vi "UI.vi"(0 "reference in":refnum<class "GUI Test Channels.lvclass">, 5 "error in (no error)":errorcluster) -> (14 "reference out":refnum<class "GUI Test Channels.lvclass">, 19 "error out":errorcluster)   [LabVIEW 2019, in "GUI Test Channels.lvclass"]
uses:
  GUI Test Channels.lvclass
  C:/Users/ANENKOV_V1/Desktop/src/GUI_class/GUI.lvclass
  FPGA/TypeDef/valveState.ctl
  GUI_class/GUI.lvclass/GUI.ctl
  TypeDef/AI_Data_Array.ctl
  TypeDef/AI_Data.ctl
  TypeDef/AI Statistics Data.ctl
  TypeDef/CalibrationData.ctl
  TypeDef/GUI Setting Channel.ctl
  TypeDef/GUI AI Ranges.ctl
  TypeDef/Scale Data.ctl
  SV_Wrap/SharedVariableWrapper.lvclass/SharedVariableWrapper.ctl
  GUI_class/WindowsState.ctl
  Modbus_class/CMD REG.ctl
  MessageAMC_class/MessageAMC.lvclass
  C:/Users/ANENKOV_V1/Desktop/src/MessageInterface_class/MessageInterface.lvclass
  147e0478-b1e0-44e5-9d90-55d61f62186e.vi
  3e1616dc-8ade-4f65-a997-ed519c35ad68.vi
  1b4fed76-272f-4eb9-b435-1b7916789d73.vi
  d0ca9bf2-7cd9-4c29-a03d-de1c10393a74.vi
  00986001-a254-421c-85fc-d87d850abbb1.vi
  b472a263-1974-420a-8762-279f74d744f3.vi
  7d6317b3-a4cc-487a-a191-d3b197fe0ad7.vi
  7b67f280-2cf4-4c83-93bd-a4bebb40b904.vi
  89ddd393-c331-4ab8-9870-c63a9689f0e3.vi
  816f4990-c02c-40e3-a8e1-ec1953188256.vi
  6ecfee0b-d9cc-4678-92a9-30749ce547e6.vi
  770577dd-3d58-4cb1-b26a-92b56a3dc732.vi
  e7cb1b03-de9d-4d10-b03f-ed147f3d7f4d.vi
  4124e316-6eb4-42ff-9d4a-b566f3345d57.vi
  b80a7f44-ff74-4897-ae94-348c9bf1cb3c.vi
  666d2444-51b8-4c74-bb7d-b80a48b6443e.vi
  GUI_class/Set Win State.vi
  147e0478-b1e0-44e5-9d90-55d61f62186e.vi/52dffe28-1cd0-4ae0-8363-fbbc473a3346.vi
  SV_Wrap/Write Var Info.vi
  SV_Wrap/Read Var Info.vi
  1b4fed76-272f-4eb9-b435-1b7916789d73.vi/5389994d-5541-411f-974c-94a5d08bd79d.vi
  d0ca9bf2-7cd9-4c29-a03d-de1c10393a74.vi/e242b2b1-b066-4fef-9774-8e1a54e29692.vi
  00986001-a254-421c-85fc-d87d850abbb1.vi/269d6d4e-e5f8-46fa-b5a0-5745950f586b.vi
  b472a263-1974-420a-8762-279f74d744f3.vi/f9a62cb2-ec71-4724-a147-a33e2b02a7cc.vi
  7d6317b3-a4cc-487a-a191-d3b197fe0ad7.vi/0852bef6-d0ca-4adc-9038-96861f44a805.vi
  7b67f280-2cf4-4c83-93bd-a4bebb40b904.vi/a928b4cf-f8d6-4ce5-931e-e4c32b09a882.vi
  89ddd393-c331-4ab8-9870-c63a9689f0e3.vi/67eb750a-c2db-4242-8b04-f1964937678c.vi
  e7cb1b03-de9d-4d10-b03f-ed147f3d7f4d.vi/e2f146e0-dd5e-45e4-842e-c2408875ec0c.vi
  SV_Wrap/Read connection str.vi
  <userlib>/_OpenG.lib/time/time.llb/Tick Count (ms)__ogtk.vi
  GUI_class/GUI.lvclass
  MessageInterface_class/MessageInterface.lvclass
  SV_Wrap/SharedVariableWrapper.lvclass
panel:
  out "CHMBR":cluster{"scl mean 1Hz":dbl, "scl mean":dbl}(graph) caption="Давление в камере [МПа]"
  out "DUT":cluster{"scl mean 1Hz":dbl, "scl mean":dbl}(graph) caption="Давление в образце [МПа]"
  out "P_CHMBR_MB":dbl caption="MB" format="%.2f"
  out "P_DUT_MB":dbl caption="MB" format="%.2f"
  in  "=0":bool
  in  "-0,1":bool
  in  "+0,1":bool
  in  "alarm press":bool
  out "data out 2":T1
  out "data out":T1
  out "AI4":dbl(slide) caption="AI 4" scale=0.0..1.0
  out "AI1":dbl(slide) caption="Температура [AI1]" scale=0.0..100.0
  out "AI3":dbl(slide)=57.25190839694657 caption="Температура [AI3]" scale=0.0..100.0
  out "AI_2":dbl(slide)=57.25190839694657 caption="Уровень [AI2]" scale=0.0..100.0
  out "AI_0":dbl(slide)=57.25190839694657 caption="Уровень [AI0]" scale=0.0..100.0
  in  "DO 25":bool caption="Stop SD [37.2]"
  in  "DO 24":bool caption="Stop SD [37.1]"
  out "DI 30":bool caption="44.2 закрыт"
  out "DI 29":bool caption="44.2 открыт"
  out "DI 22":bool caption="44.1 закрыт"
  out "DI 21":bool caption="44.1 открыт"
  in  "DO 23":bool caption="KP24 Y44.2 抢市."
  in  "DO 22":bool caption="KP23 Y44.2 ОТК."
  in  "DO 21":bool caption="KP22 Y44.1 抢市."
  in  "DO 20":bool caption="KP21 Y44.1 ОТК."
  in  "DO 19":bool caption="Драйверы KP20"
  in  "DO 17":bool caption="KP18 Y29.13 33.3"
  in  "DO 18":bool caption="Подача воздук KP19"
  out "DI 11":bool caption="Состояние БП [G2]"
  out "DI 20":bool caption="Фильтр [S4]"
  out "DI 19":bool caption="Фильтр [S3]"
  out "DI 18":bool caption="Фильтр [S2]"
  out "DI 17":bool caption="Фильтр [S1]"
  out "DI 8":bool caption="QF9"
  out "DI 7":bool caption="QF8"
  out "DI 6":bool caption="QF7"
  out "DI 5":bool caption="QF6"
  out "Connect":bool caption="Подключение"
  in  "Reset Alarms":bool
  in  "stop":bool
  out "DI 10":bool caption="Состояние БП [G1]"
  out "DI 9":bool caption="Реле контроля фаз, контактор [KV1]"
  out "DI 4":bool caption="QF5"
  out "DI 3":bool caption="QF4"
  out "DI 2":bool caption="QF3"
  out "DI 1":bool caption="QF2"
  out "DI 0":bool caption="QF1"
  out "DI 26":bool caption="Автомат [QF12]"
  out "DI 25":bool caption="Контактор [MK2]"
  out "DI 28":bool caption="Автомат [QF13]"
  out "DI 27":bool caption="Контактор [MK3]"
  out "DI 24":bool caption="Автомат [QF11]"
  out "DI 23":bool caption="Контактор [MK1]"
  in  "AO 1":dbl(slide) caption="AO 0" scale=0.0..10.0
  in  "AO 0":dbl(slide) min=0.0 max=2.0 step=0.01 scale=0.0..1.0 scale format="%#.2f"
  in  "DO 16":bool caption="KP17 Y29.12  33.4"
  in  "DO 15":bool caption="KP16 Y29.11  33.5"
  in  "DO 14":bool caption="KP15 Y29.10  33.6"
  in  "DO 13":bool caption="KP14 Y29.9 33.10"
  in  "DO 12":bool caption="KP13 Y29.8  33.11"
  in  "DO 11":bool caption="KP12 Y29.7  33.13"
  in  "DO 10":bool caption="KP11 Y29.6 33.2"
  in  "DO 9":bool caption="KP10 Y29.5 33.1"
  in  "DO 8":bool caption="KP9 Y29.4  33.12"
  in  "DO 7":bool caption="KP8 Y29.3 33.9"
  in  "DO 6":bool caption="KP7 Y29.2 33.8"
  in  "DO 5":bool caption="KP6 Y29.1 33.7"
  in  "DO 4":bool caption="Вода Y18.2 [DO4]"
  in  "DO 3":bool caption="Вода Y18.1 [DO3]"
  in  "DO 2":bool caption="Пуск KP3 [DO 2]"
  in  "DO 1":bool caption="Пуск KP2 [DO 1]"
  in  "DO 0":bool caption="Пуск KP1 [DO 0]"
  out "DI 16":bool caption="Переключатель ручное/авто SA1"
  out "DI 15":bool caption="Кнопка аварийной остановки [SB4]"
  out "DI 14":bool caption="Кнопка остановки [SB3]"
  out "DI 13":bool caption="Кнопка запуска [SB2]"
  out "DI 12":bool caption="Кнопка сброса ошибки [SB1]"
  out "AI 10":dbl(knob) caption="Датчик давления в линии \nизмерения утечек  [бар]" scale=0.0..400.0
  out "AI 9":dbl(knob) caption="Давление  в  линии подачи \nвоздуха после БПВ [бар]" scale=0.0..16.0
  out "AI 8":dbl(knob) caption="Давление  в  линии подачи \nвоздуха в БПВ  [бар]" scale=0.0..16.0
  out "AI 7":dbl(knob) caption="Давление в камере [МПа]" scale=0.0..400.0
  out "AI 6":dbl(knob) caption="Давление в образце [МПа]" scale=0.0..400.0
  out "AI 5":dbl(knob) caption="Давление после насоса ВД [МПа]" scale=0.0..400.0
  # "Проверка каналов"
  # "Панель гидравлическая"
  # "Кнопки"
  # "Реле"
  # "Гидростанция очистки и охлаждения [M24]"
  # "Насос перекачки \nв бак подачи [M12]"
  # "Автоматы"
  # "Гидростанция подачи масла [M21]"
  # "Управление  подачей давления в насос ВД"
  # "Регулировка низкого давления в линии подачи масла в насос ВД и напрямую в узел образца"
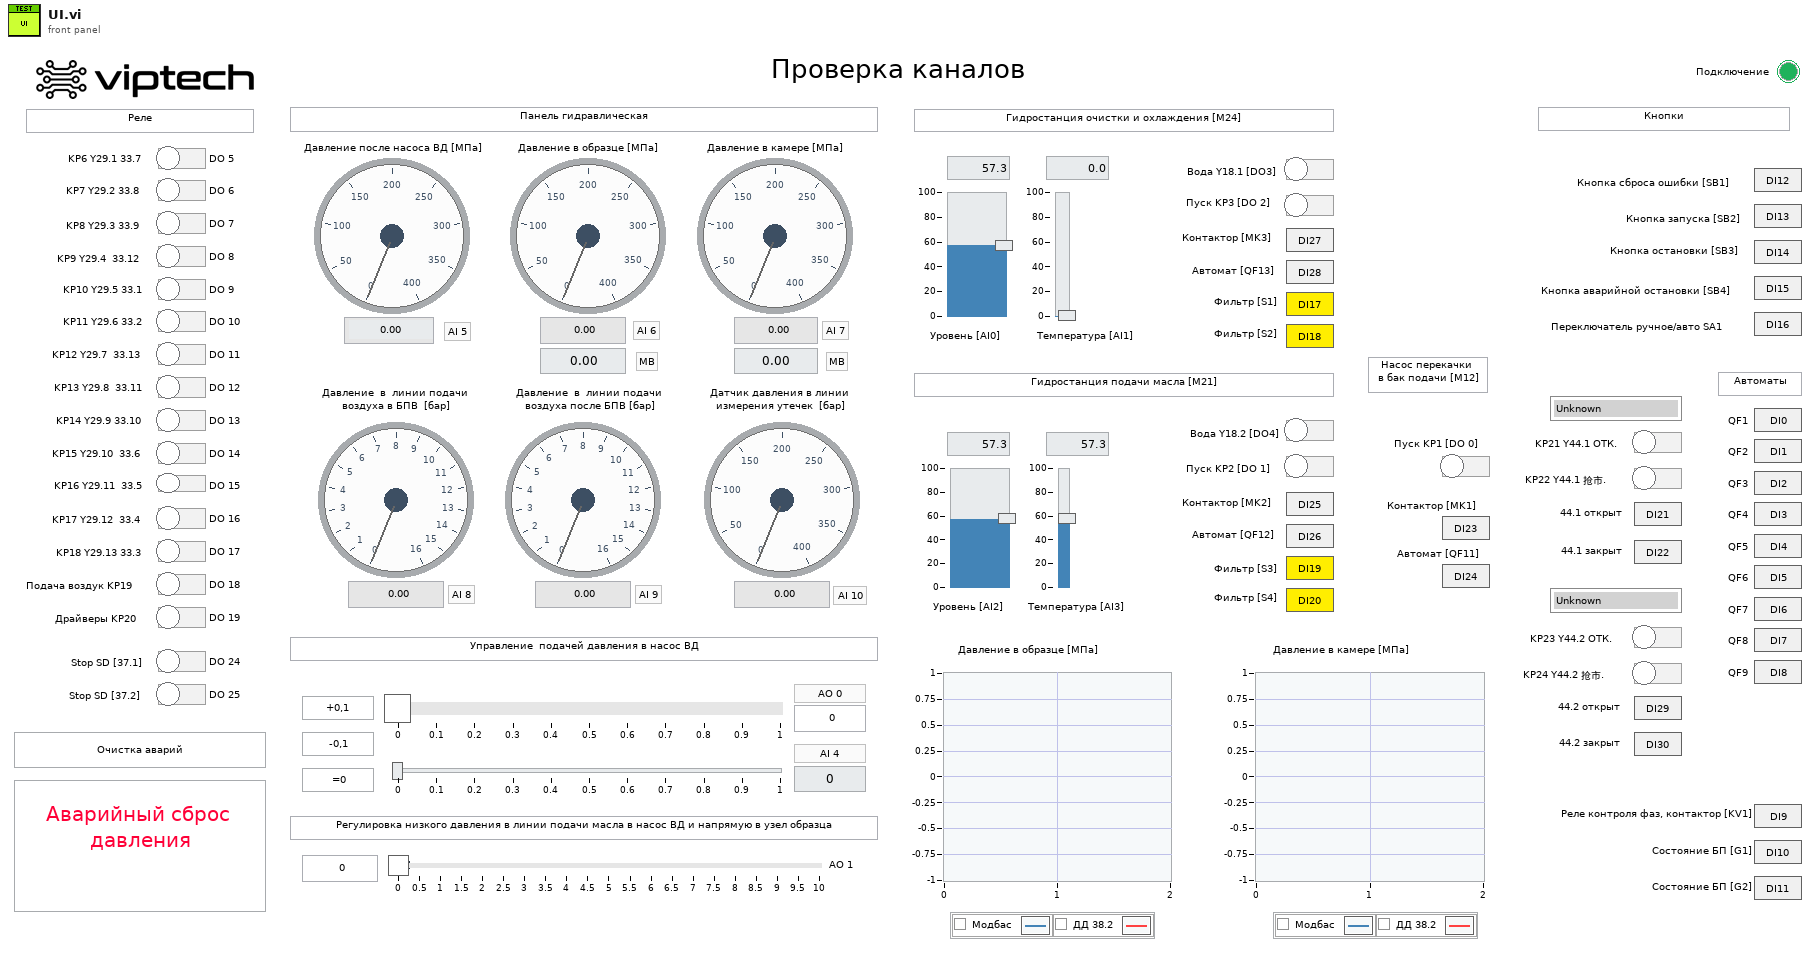
[diagram p1: front panel]
types:
  T1 = typedef "valveState.ctl" = enum16{"Unknown", "Closed", "Opening", "Opened", "Closing"}
  T2 = typedef "CMD REG.ctl" = cluster{"EXECUTE_SP":bool, "ALARM_PRESS_DOWN_DUT":bool, "ALARM_PRESS_DOWN_CHAMBER":bool, "ALARM_PRESS_DOWN_DUT_CHAMBER":bool, "FILING_DUT":bool, "FILING_CHAMBER":bool, "BLOCK":bool, "PUMP_STATION_OFF":bool, "Leak start":bool, "Leak stop":bool, "Drain":bool}
  T3 = enum32{"Invalid", "Standard", "Closed", "Hidden", "Minimized", "Maximized"}
  T4 = enum32{"invalid app kind", "Development System", "Run Time System", "Student Edition", "Embedded LabVIEW", "Evaluation", "Custom"}
  T5 = typedef "SharedVariableWrapper.lvclass/Config.ctl" = cluster{"connection str":string, "timeout":dbl, "ip":string}
  T6 = cluster{"Core":cluster{"Current VI Reference":refnum<vi>, "Close Panel on Exit?":bool}, "amc":refnum<class "MessageAMC.lvclass">}
  T7 = cluster{"Current VI Reference":refnum<vi>, "Close Panel on Exit?":bool}
  T8 = typedef "CalibrationData.ctl" = cluster{"Channels":T9[], "Scales":T11[]}
  T9 = typedef "GUI Setting Channel.ctl" = cluster{"Name":string, "AI Ranges":T10, "ScaleIndex":u32}
  T10 = typedef "GUI AI Ranges.ctl" = cluster{"HI":bool, "HIHI":bool, "LO":bool, "LOLO":bool, "HIHI VAL":dbl, "HI VAL":dbl, "LO VAL":dbl, "LOLO VAL":dbl, "MAX RAW":dbl, "MIN RAW":dbl, "MAX SCALED":dbl, "MIN SCALED":dbl}
  T11 = typedef "Scale Data.ctl" = cluster{"index":i32, "Name":string, "X":dbl[], "Y":dbl[]}
  T12 = typedef "AI_Data_Array.ctl" = T13[]
  T13 = typedef "AI_Data.ctl" = cluster{"Stat Data":T14, "OutOfRangeMax":bool, "OutOfRangeMin":bool, "HIHI":bool, "HI":bool, "LO":bool, "LOLO":bool}
  T14 = typedef "AI Statistics Data.ctl" = cluster{"raw mean":dbl, "scl mean":dbl, "raw mean 1Hz":dbl, "scl mean 1Hz":dbl}
  T15 = typedef "GUI.lvclass/WindowsState.ctl" = enum16{"NotReady", "Ready", "Inserted", "Opened"}
  T16 = typedef "GUI.lvclass/Shered Data.ctl" = cluster{"WindowsState":T15, "UI VI":refnum<vi>, "SubPnl":refnum<vi>}
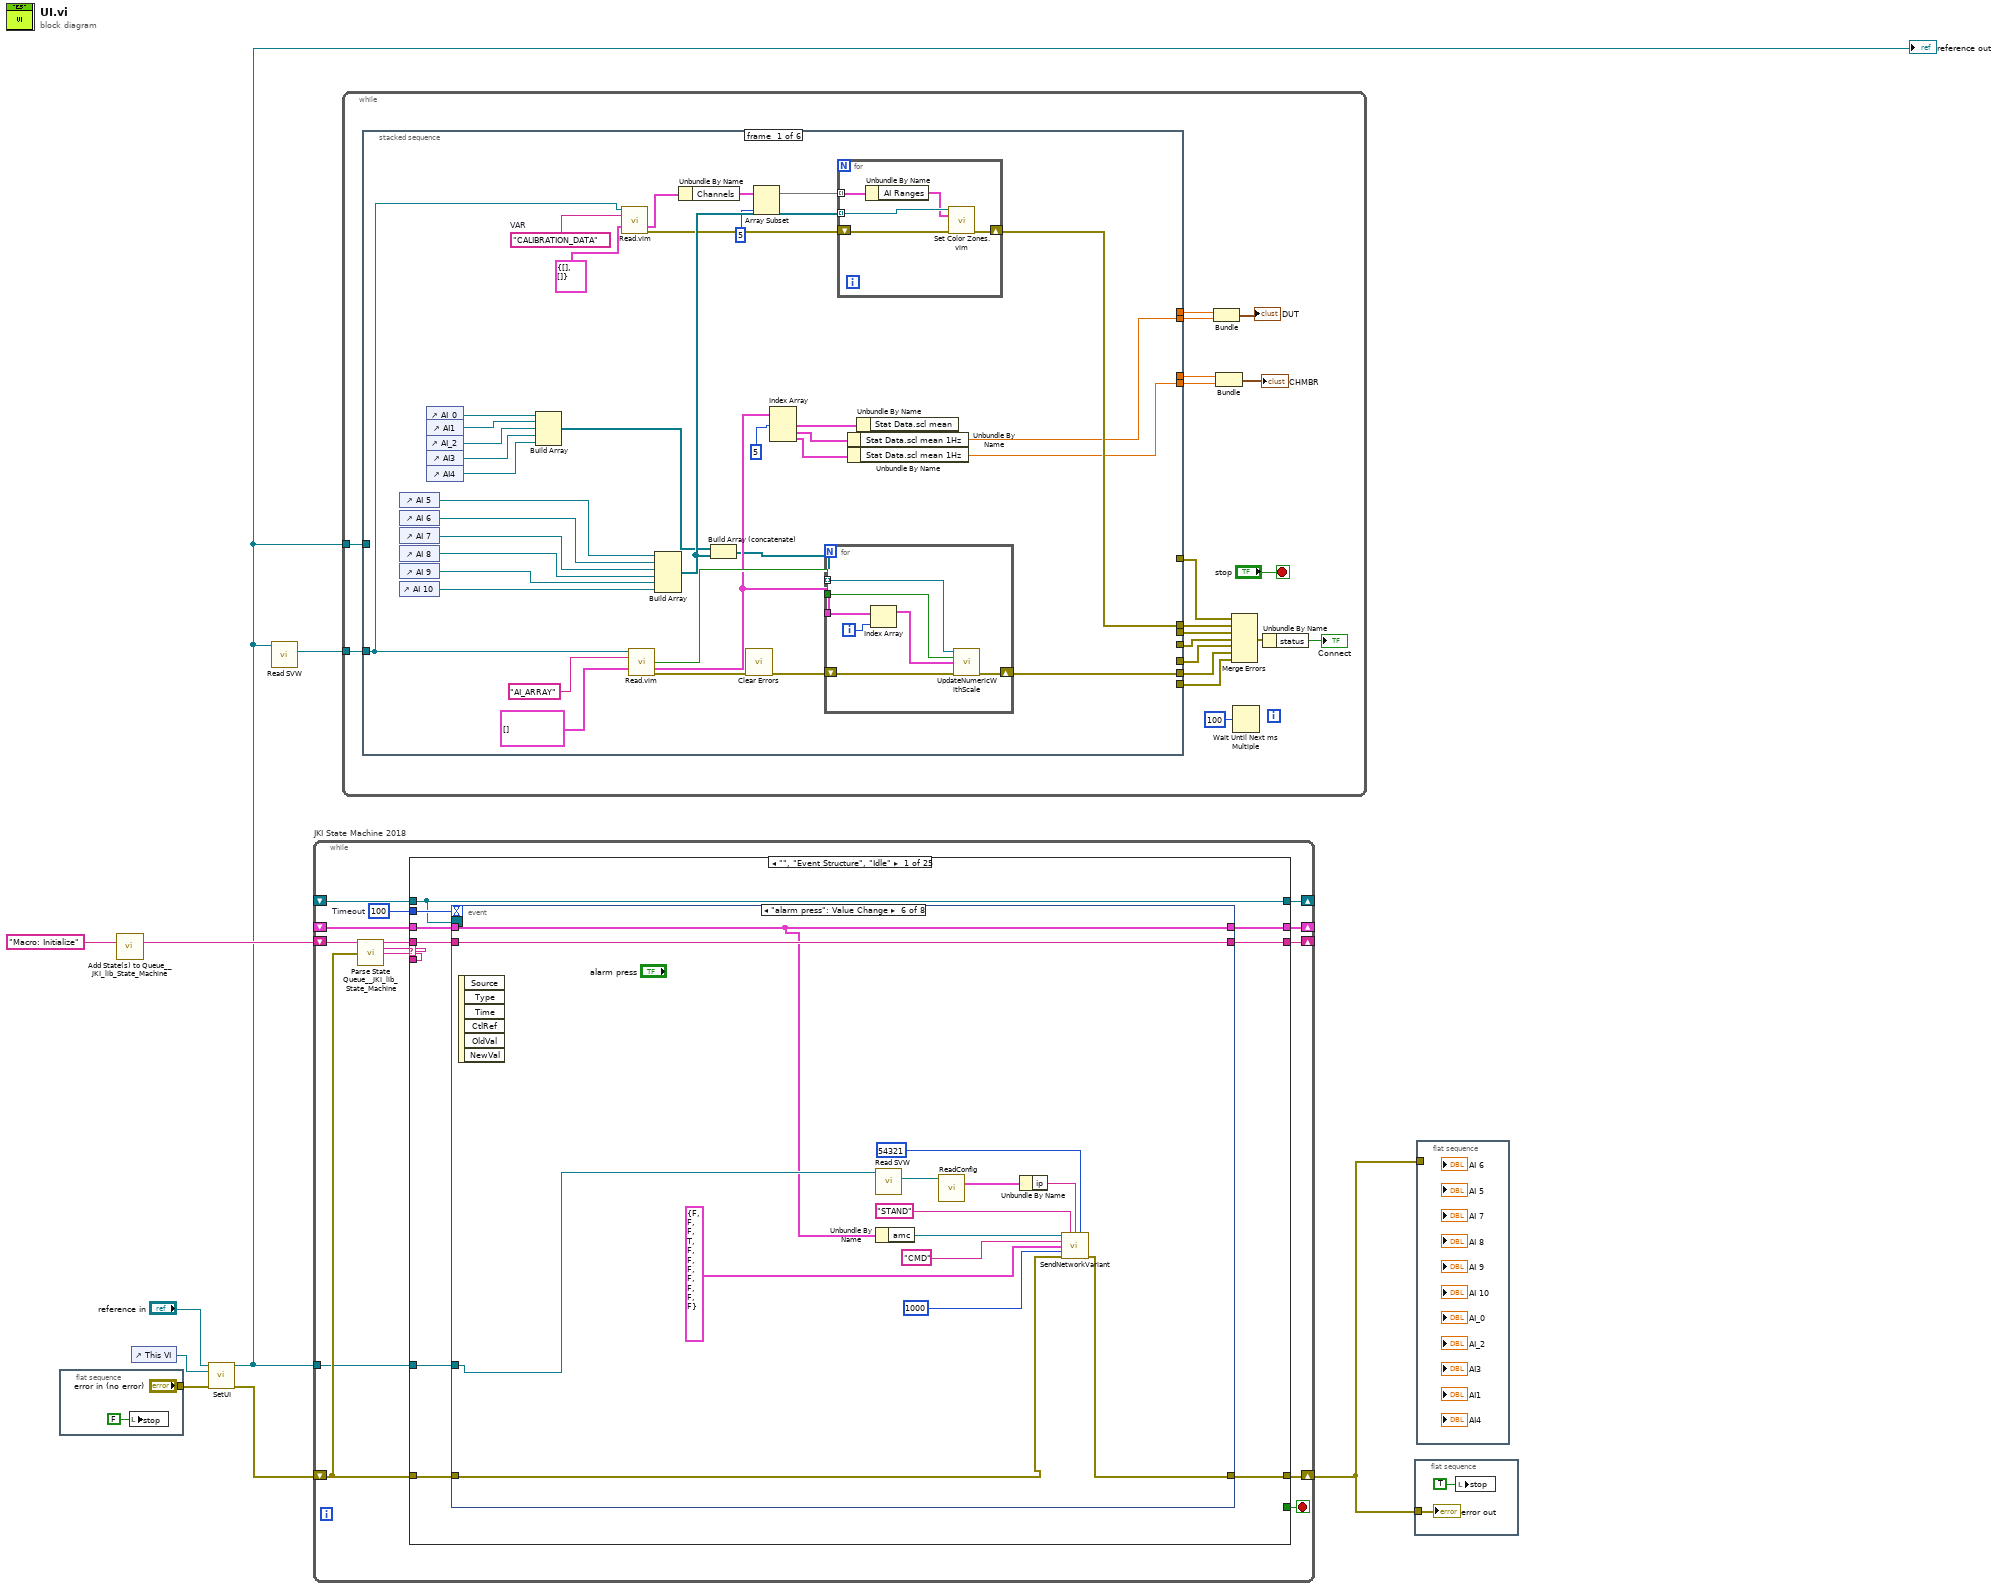
[diagram p0: block diagram]
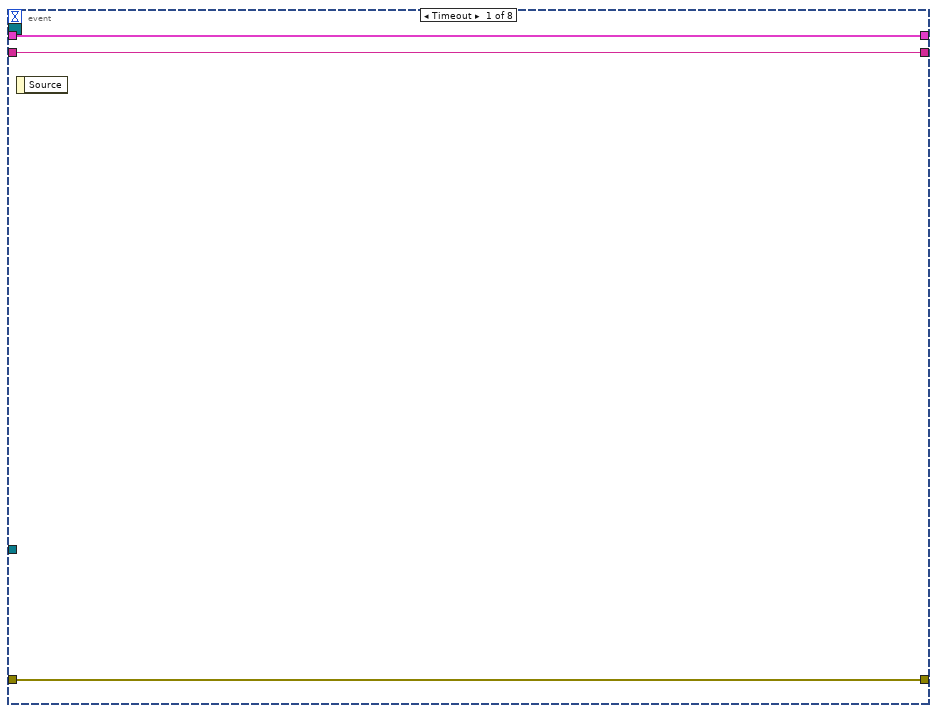
[diagram p2: hidden frame]
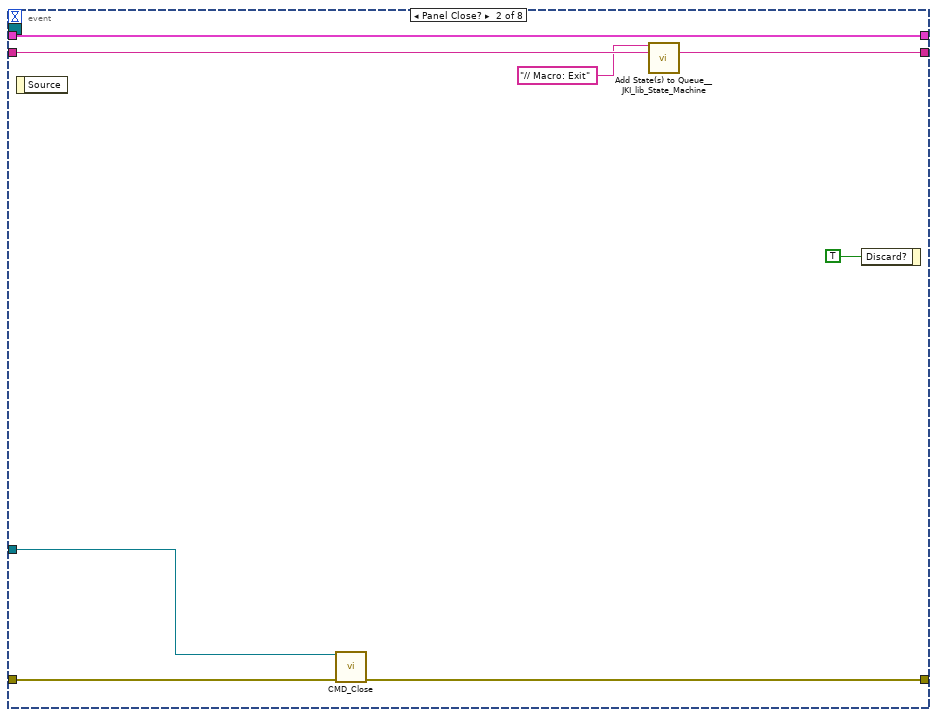
[diagram p3: hidden frame]
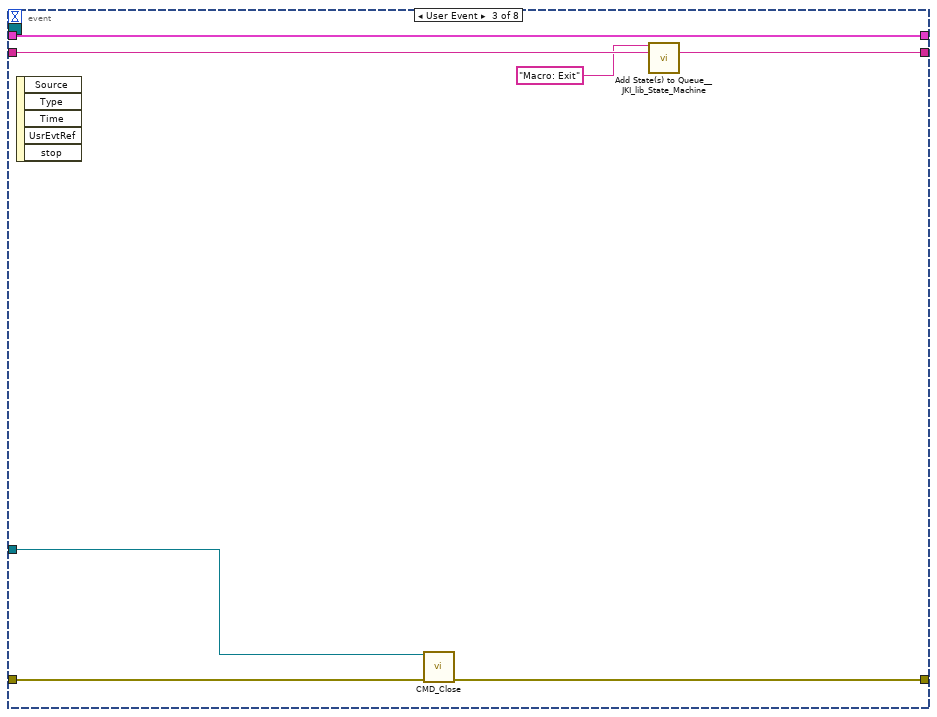
[diagram p4: hidden frame]
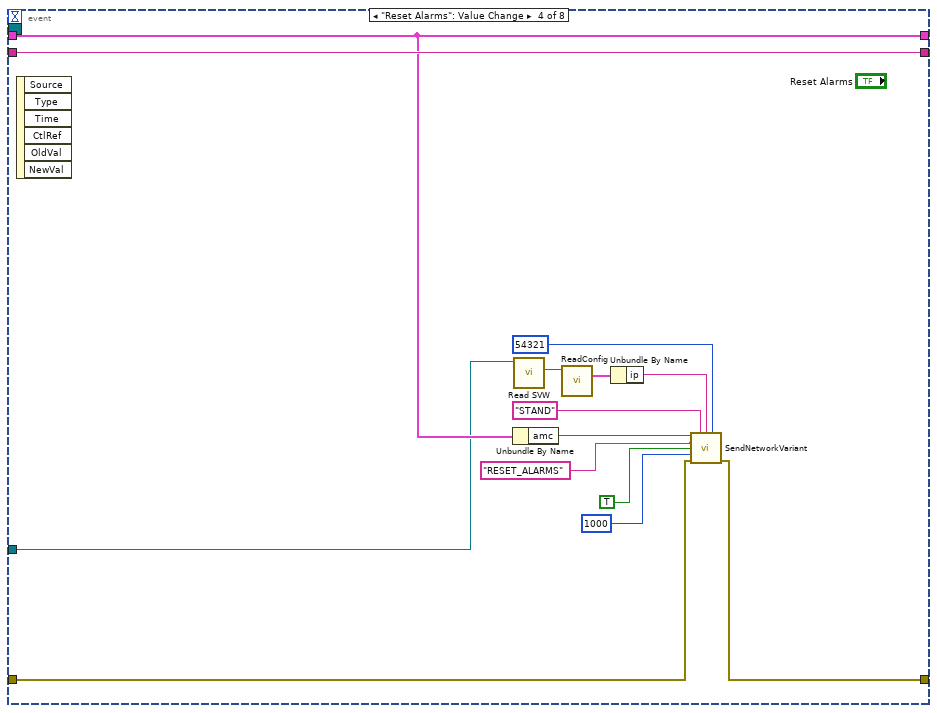
[diagram p5: hidden frame]
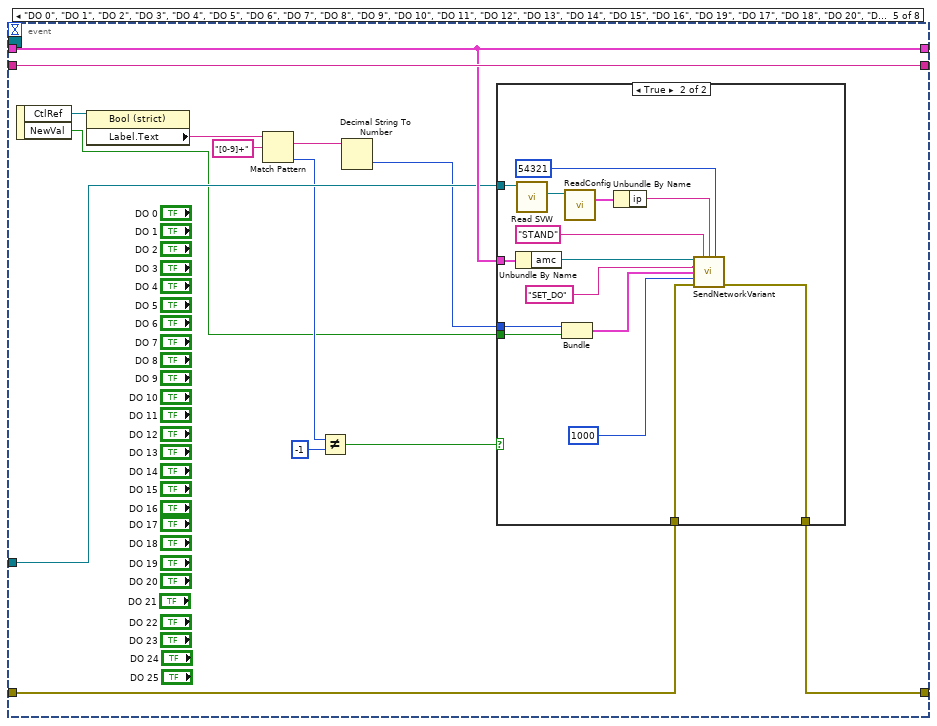
[diagram p6: hidden frame]
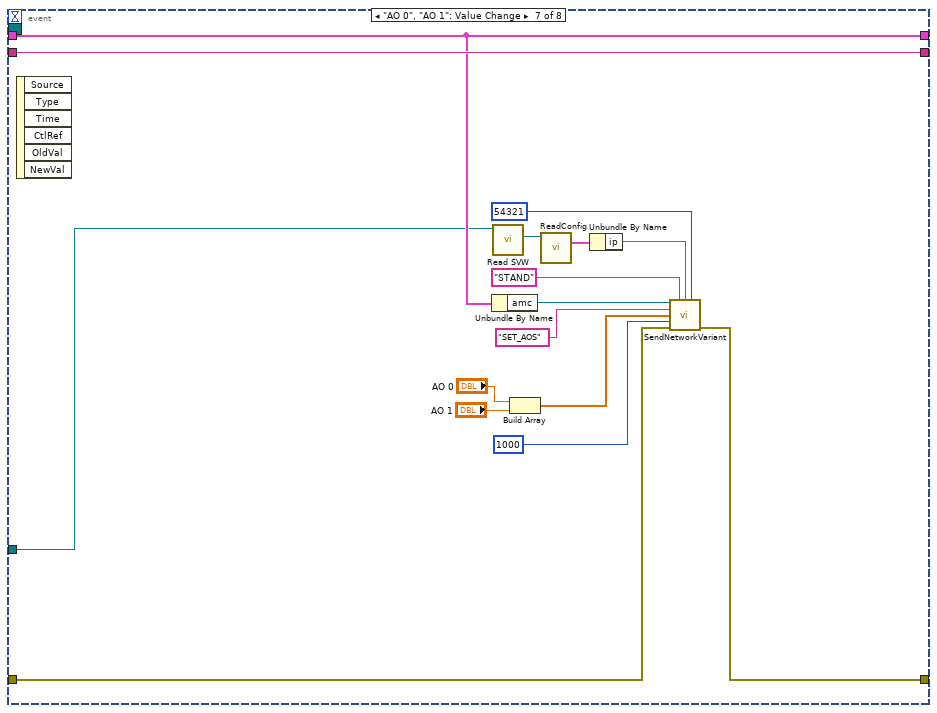
[diagram p8: hidden frame]
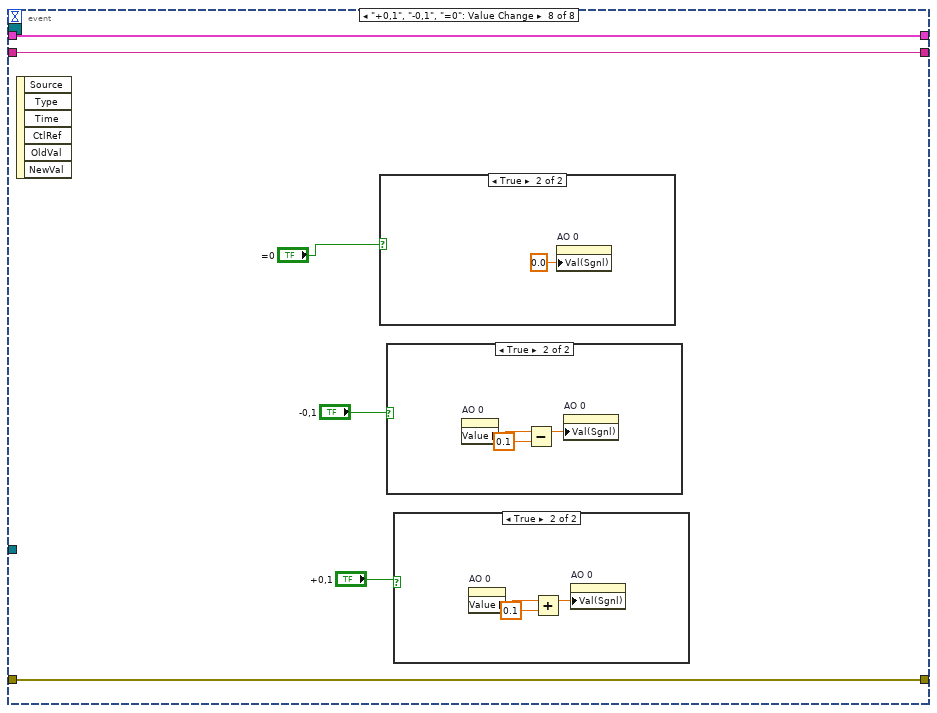
[diagram p9: hidden frame]
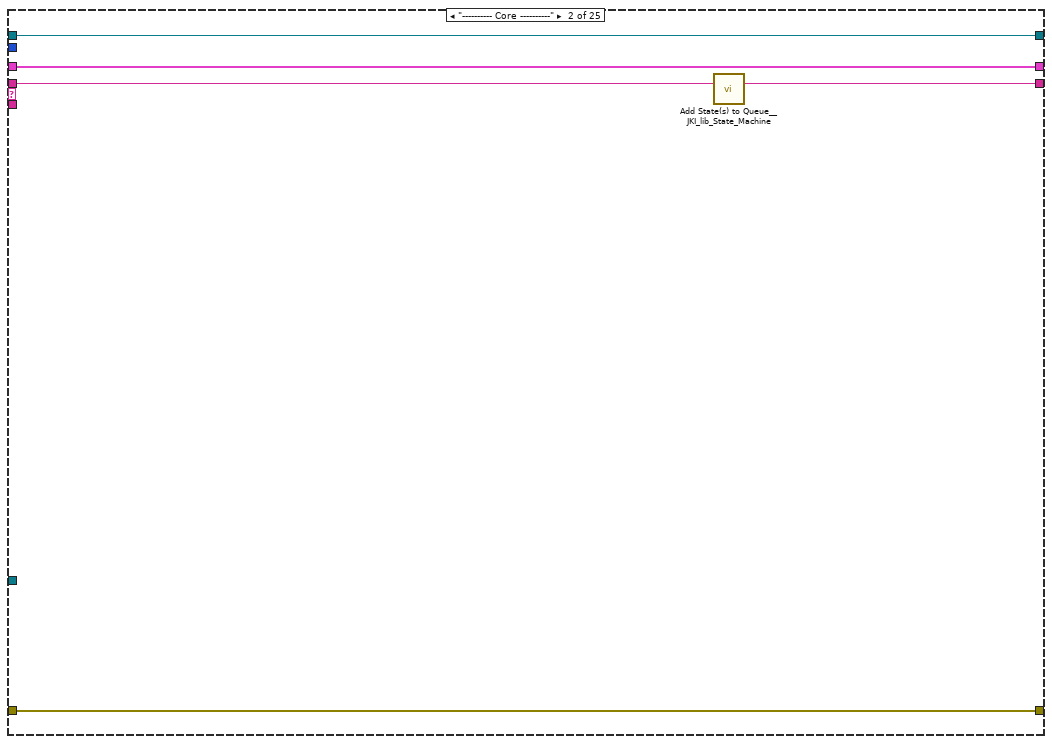
[diagram p13: hidden frame]
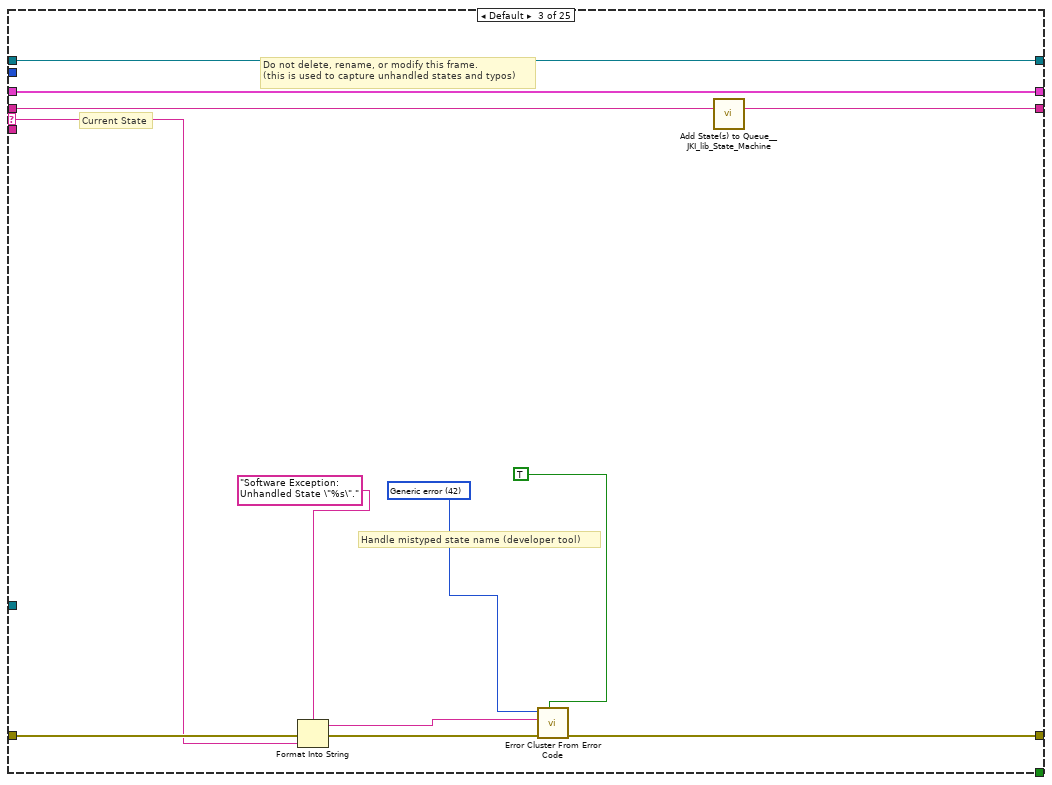
[diagram p14: hidden frame]
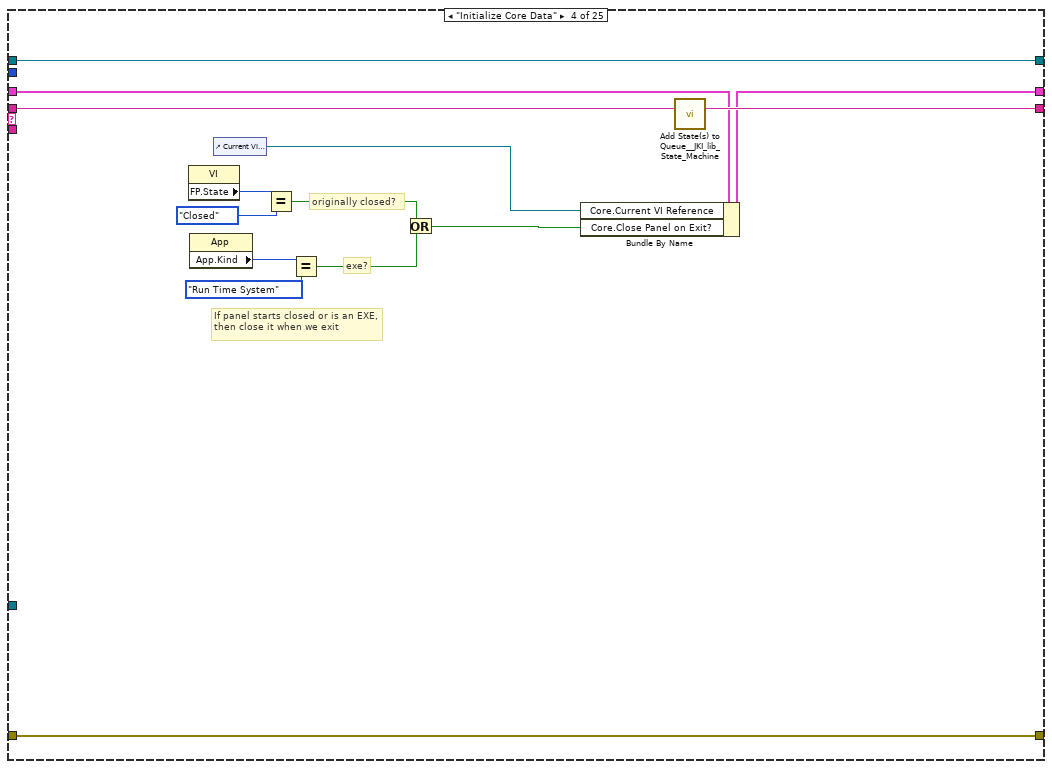
[diagram p15: hidden frame]
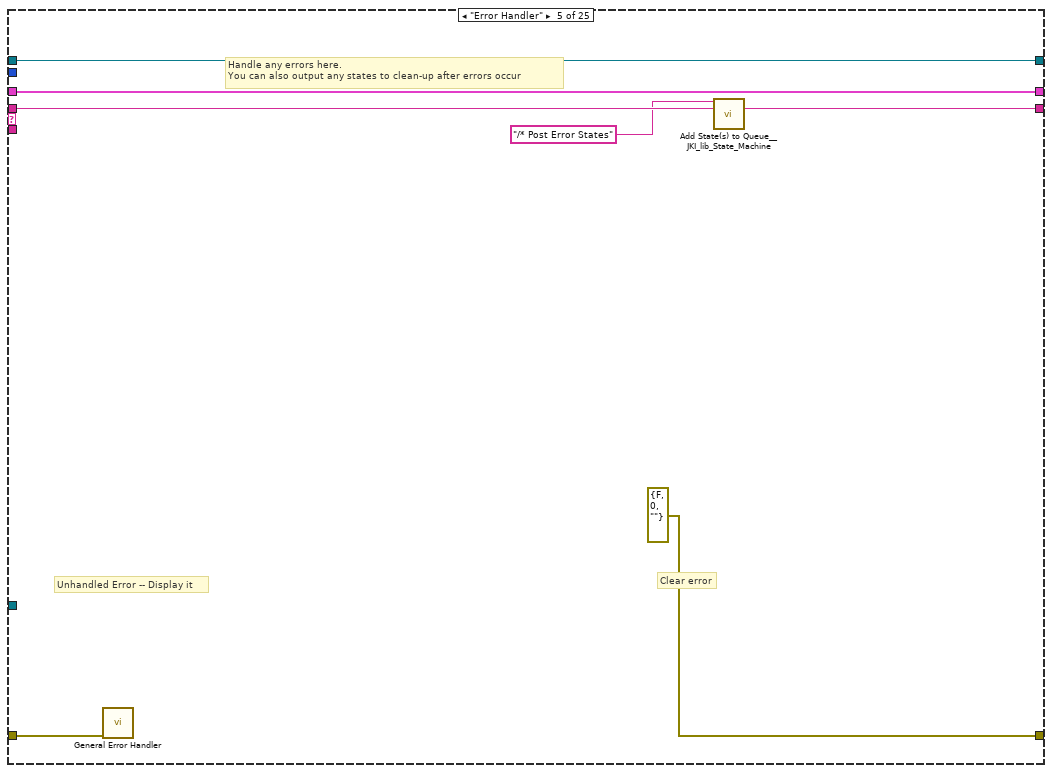
[diagram p16: hidden frame]
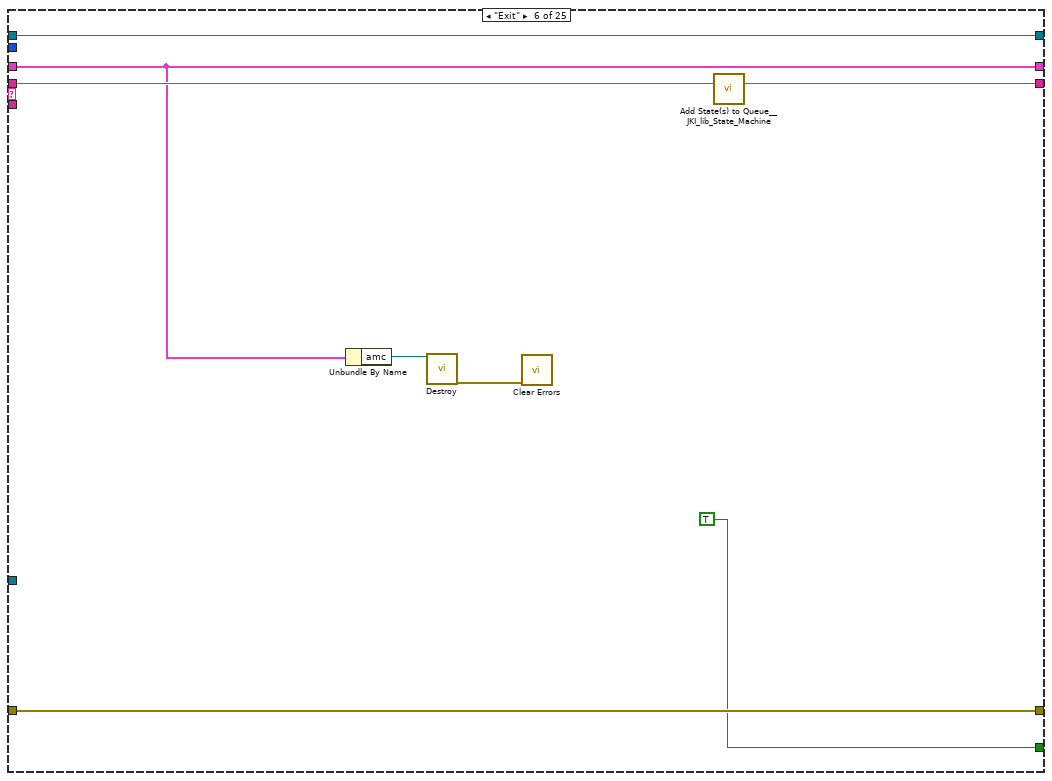
[diagram p17: hidden frame]
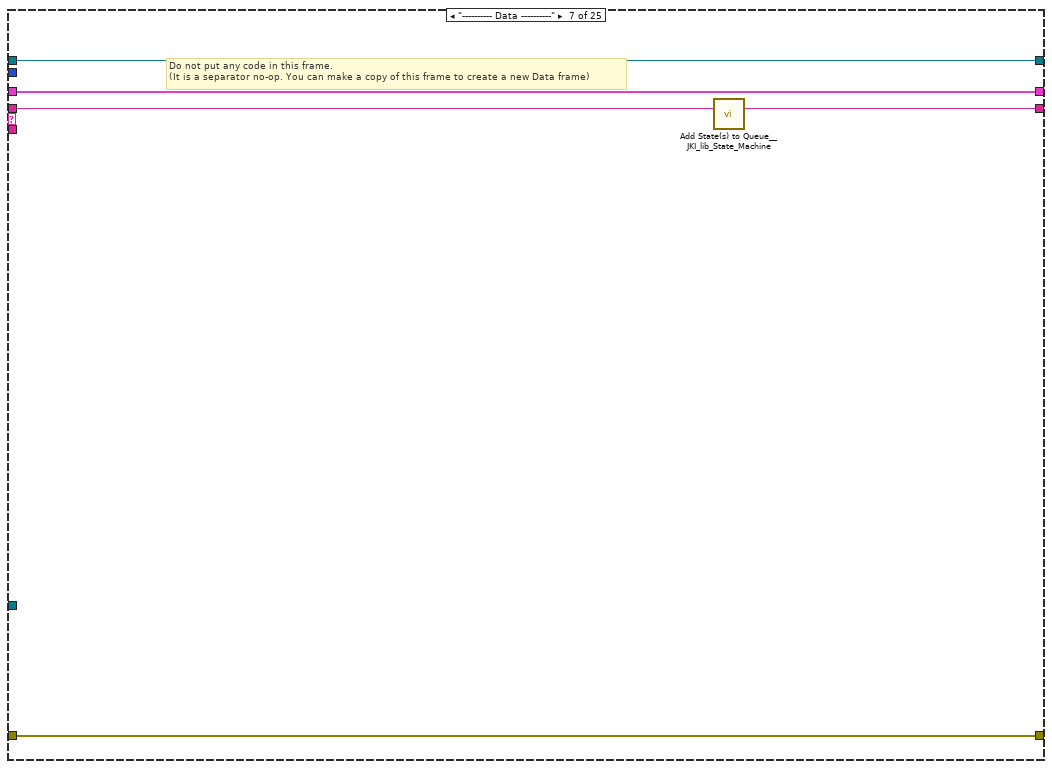
[diagram p18: hidden frame]
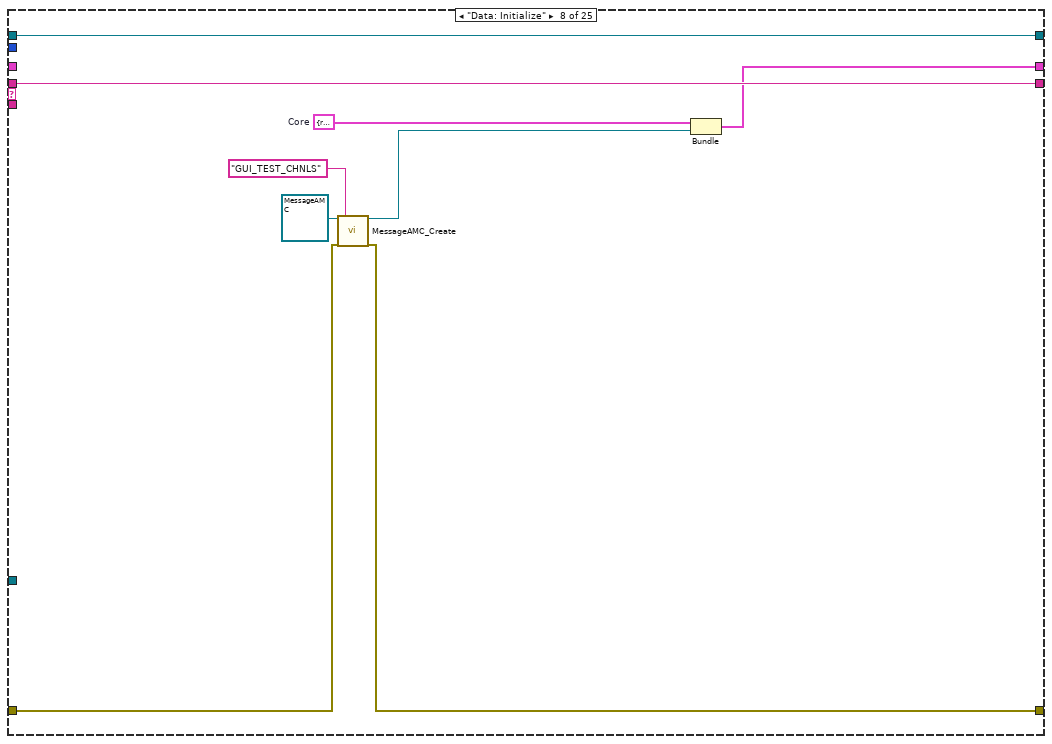
[diagram p19: hidden frame]
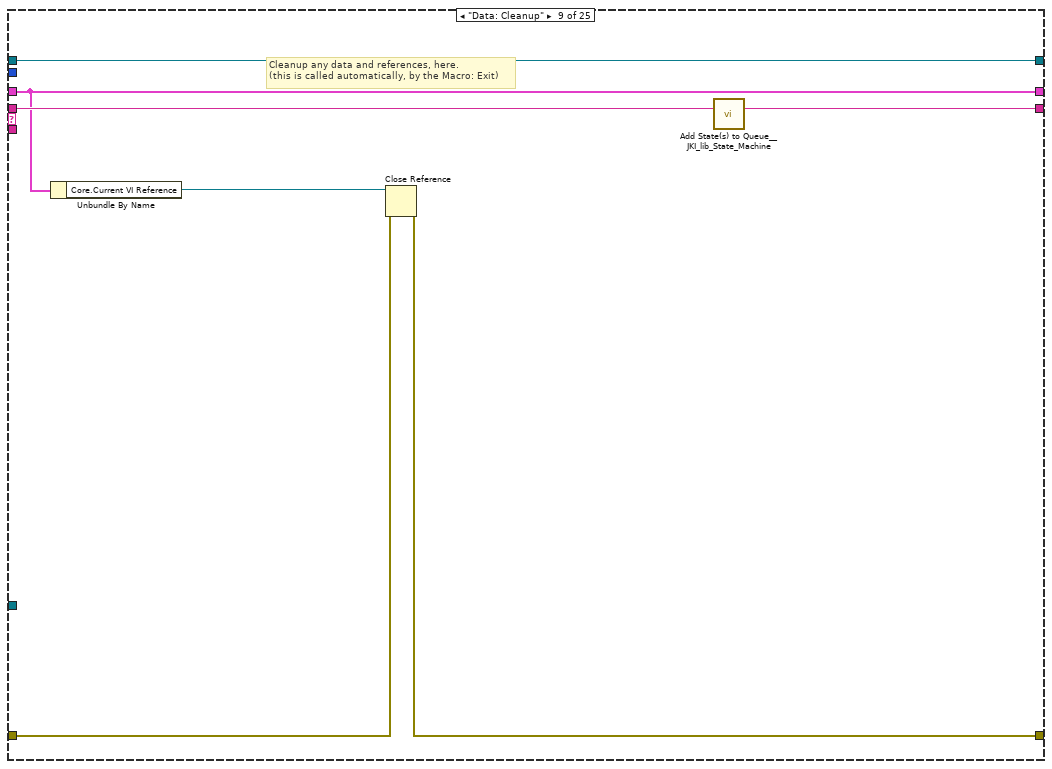
[diagram p20: hidden frame]
diagram:
  n1 = flat-sequence {
    tunnel: ["error in (no error)"] -> w7
    frame #0 {
      n2 = local write "stop"(FALSE ("stop")) -> ()
    }
  }
  n3 = call <vilib>:"Add State(s) to Queue__JKI_lib_State_Machine.vi"("State(s) in (\"\")"="Macro: Initialize") -> ("States Out"=w9:string)  [unwired: 14 in]
  n4 = control-ref of="This VI"() -> (w5:refnum<vi>)
  n5 = call "SetUI.vi"("reference in"="reference in", "UI VI"=w5, "error in (no error)"=w7) -> ("reference out"=w2:refnum<class "GUI Test Channels.lvclass">, "error out"=w4:errorcluster)  [unwired: 11 in]
  "reference out" <- w2
  n6 = call "Read SVW.vi"("GUI in"=w2) -> ("SharedVariableWrapper.lvclass"=w3:refnum<class "SharedVariableWrapper.lvclass">)  [unwired: 10 in]
  n7 = while "JKI State Machine 2018" {
    shift-right: [w18] -> _
    shift-left: _ -> [w17]
    shift-right: [w21] -> w1
    shift-left: w4 -> [w15]
    shift-right: [w20] -> _
    shift-left: w9 -> [w22]
    tunnel: w2 -> [w14]
    shift-right: [w13] -> _
    shift-left: _ -> [w12]
    stop <- w19 stop-if-true
    w16 = 100  # Timeout
    n8 = call <vilib>:"Parse State Queue__JKI_lib_State_Machine.vi"("State Queue"=w22, "Error In (no error)"=w15) -> ("Remaining States"=w24:string, "Current State"=w25:string, "Arguments"=w23:string)  [unwired: 11 in]
    n9 = case shown="\"\", \"Event Structure\", \"Idle\"" w25 {
      selector: w25 -> [_ _ w146 _ _ _ _ _ _ _ _ _ _ _ _ _ _ _ _ _ _ _ _ _ _]
      tunnel: w24 -> [w34 w144 w150 w170 w177 w185 w190 w199 w206 w211 w218 w224 w229 w233 w240 w252 w322 w328 w334 w346 w350 w351 w359 w363 w365]
      tunnel: w23 -> [_ _ _ _ _ _ _ _ _ _ _ _ _ _ w235 w246 _ _ _ _ _ _ _ _ _]
      tunnel: w17 -> [w32 w141 w148 w163 w174 w180 w187 _ w201 w208 w217 w222 w226 w232 w238 w248 w319 w325 w331 w343 w348 w353 w357 w360 w364]
      tunnel: [w31 w142 w152 w167 errorcluster {"status"=FALSE, "code"=0, "source"=""} ("error out") w183 w188 w192 w202 w209 w215 w219 w227 w231 w236 w249 w320 w326 w332 w344 w349 w354 w356 w361 w367] -> w21
      tunnel: w15 -> [w30 w142 w151 w167 w173 w183 w188 w193 w203 w209 w214 w220 w227 w231 w237 w250 w320 w326 w332 w344 w349 w354 w356 w361 w367]
      tunnel: [w33 w143 w149 w169 w176 w184 w189 w199 w205 w210 w218 w223 w228 w233 w239 w251 w321 w327 w333 w345 w350 w352 w359 w363 w365] -> w20
      tunnel: [_ _ _ _ _ TRUE _ _ _ _ _ _ _ _ _ _ _ _ _ _ _ _ _ _ _] -> w19
      tunnel: [w29 w141 w148 w168 w174 w180 w187 w198 w201 w208 w217 w222 w226 w232 w238 w248 w319 w325 w331 w343 w348 w353 w357 w360 w364] -> w18
      tunnel: w16 -> [w28 _ _ _ _ _ _ _ _ _ _ _ _ _ _ _ _ _ _ _ _ _ _ _ _]
      tunnel: w14 -> [w27 _ _ _ _ _ _ _ _ _ w213 _ _ _ _ _ _ _ _ _ _ _ _ _ _]
      tunnel: [w26 w140 w145 w157 w171 w181 w186 w196 w200 w207 w216 w221 w225 w230 w234 w245 w318 w323 w329 w336 w347 w355 w358 w362 w366] -> w13
      tunnel: w12 -> [w26 w140 w145 w157 w171 w181 w186 w196 w200 w207 _ w221 w225 w230 w234 w245 w318 w323 w329 w336 w347 w355 w358 w362 w366]
      frame "", "Event Structure", "Idle" {
        n10 = event shown="[5] \"alarm press\": Value Change" {
          selector: w26 -> [_ _ _ _ _ _ _ _]
          dyn-events: _ -> [_ _ _ _ _ _ _ _]
          timeout: w28 -> [_ _ _ _ _ _ _ _]
          tunnel: w34 -> [w37 w45 w52 w66 w80 w110 w126 w132]
          tunnel: [w37 w44 w51 w66 w80 w110 w126 w132] -> w33
          tunnel: w32 -> [w35 w43 w50 w56 w79 w99 w114 w130]
          tunnel: [w36 w38 w46 w57 w76 w97 w111 w131] -> w31
          tunnel: w30 -> [w36 w39 w47 w55 w77 w98 w112 w131]
          tunnel: [w35 w43 w50 w56 w79 w99 w114 w130] -> w29
          tunnel: w27 -> [_ w40 w48 w53 w78 w100 w113 _]
          event Timeout {
            n11 = event-data() -> ()  [unwired: 1 in, 1 out]
          }
          event Panel Close? {
            n12 = event-data() -> ()  [unwired: 1 in, 1 out]
            n13 = call "CMD_Close.vi"("reference in"=w40, "error in (no error)"=w39) -> ("error out"=w38:errorcluster)  [unwired: 12 in, 1 out]
            n14 = call <vilib>:"Add State(s) to Queue__JKI_lib_State_Machine.vi"("State(s) in Front (\"\")"="// Macro: Exit", "State(s) in (\"\")"=w45) -> ("States Out"=w44:string)  [unwired: 13 in]
            n15 = event-data("Discard?"=TRUE) -> ()  [unwired: 1 in, 1 out]
          }
          event User Event {
            n16 = event-data() -> ()  [unwired: 1 in, 5 out]
            n17 = call "CMD_Close.vi"("reference in"=w48, "error in (no error)"=w47) -> ("error out"=w46:errorcluster)  [unwired: 12 in, 1 out]
            n18 = call <vilib>:"Add State(s) to Queue__JKI_lib_State_Machine.vi"("State(s) in Front (\"\")"="Macro: Exit", "State(s) in (\"\")"=w52) -> ("States Out"=w51:string)  [unwired: 13 in]
          }
          event "Reset Alarms": Value Change {
            n19 = event-data() -> ()  [unwired: 1 in, 6 out]
            n20 = Unbundle By Name(w56) -> ("amc"=w65:refnum<class "MessageAMC.lvclass">)
            n21 = call "Read SVW.vi"("GUI in"=w53) -> ("SharedVariableWrapper.lvclass"=w60:refnum<class "SharedVariableWrapper.lvclass">)  [unwired: 10 in]
            n22 = call "ReadConfig.vi"("SharedVariableWrapper in"=w60) -> ("config"=w59:T5)  [unwired: 12 in, 2 out]
            n23 = Unbundle By Name(w59) -> ("ip"=w58:string)
            n24 = call "SendNetworkVariant.vi"("reference in"=w65, "receiver process"="STAND", "receiver host"=w58, "receiver port (0)"=u16 54321, "name"="RESET_ALARMS", "data"=TRUE, "timeout (25000 ms)"=1000, "error in (no error)"=w55) -> ("error out"=w57:errorcluster)  [unwired: 5 in, 2 out]
          }
          event "DO 0", "DO 1", "DO 2", "DO 3", "DO 4", "DO 5", "DO 6", "DO 7", "DO 8", "DO 9", "DO 10", "DO 11", "DO 12", "DO 13", "DO 14", "DO 15", "DO 16", "DO 19", "DO 17", "DO 18", "DO 20", "DO 21", "DO 22", "DO 23", "DO 24", "DO 25": Value Change {
            n25 = event-data() -> ("CtlRef"=w71:refnum<vi>, "NewVal"=w67:bool)  [unwired: 1 in]
            n26 = property class="Bool (strict)"(reference=w71) -> ("Label.Text"=w70:string)  [unwired: 1 in, 2 out]
            n27 = Match Pattern(string=w70, regular expression="[0-9]+") -> (match substring=w72:string, offset past match=w74:i32)  [unwired: 1 in, 2 out]
            n28 = Not Equal?(x=w74, y=-1) -> (x != y?=w69:bool)
            n29 = Decimal String To Number(string=w72) -> (number=w68:i32)  [unwired: 2 in, 1 out]
            n30 = case shown="True" w69 {
              tunnel: w79 -> [_ w96]
              tunnel: w78 -> [_ w95]
              tunnel: w77 -> [w81 w94]
              tunnel: [w81 w93] -> w76
              tunnel: w68 -> [_ w84]
              tunnel: w67 -> [_ w83]
              frame False {
              }
              frame True {
                n31 = Unbundle By Name(w96) -> ("amc"=w92:refnum<class "MessageAMC.lvclass">)
                n32 = call "Read SVW.vi"("GUI in"=w95) -> ("SharedVariableWrapper.lvclass"=w87:refnum<class "SharedVariableWrapper.lvclass">)  [unwired: 10 in]
                n33 = Bundle(w84, "NewVal"=w83) -> (w82:cluster{i32, "NewVal":bool})  [unwired: 1 in]
                n34 = call "ReadConfig.vi"("SharedVariableWrapper in"=w87) -> ("config"=w86:T5)  [unwired: 12 in, 2 out]
                n35 = Unbundle By Name(w86) -> ("ip"=w85:string)
                n36 = call "SendNetworkVariant.vi"("reference in"=w92, "receiver process"="STAND", "receiver host"=w85, "receiver port (0)"=u16 54321, "name"="SET_DO", "data"=w82, "timeout (25000 ms)"=1000, "error in (no error)"=w94) -> ("error out"=w93:errorcluster)  [unwired: 5 in, 2 out]
              }
            }
          }
          event "alarm press": Value Change {
            n37 = event-data() -> ()  [unwired: 1 in, 6 out]
            n38 = call "Read SVW.vi"("GUI in"=w100) -> ("SharedVariableWrapper.lvclass"=w109:refnum<class "SharedVariableWrapper.lvclass">)  [unwired: 10 in]
            n39 = Unbundle By Name(w99) -> ("amc"=w101:refnum<class "MessageAMC.lvclass">)
            n40 = call "ReadConfig.vi"("SharedVariableWrapper in"=w109) -> ("config"=w108:T5)  [unwired: 12 in, 2 out]
            n41 = Unbundle By Name(w108) -> ("ip"=w107:string)
            n42 = call "SendNetworkVariant.vi"("reference in"=w101, "receiver process"="STAND", "receiver host"=w107, "receiver port (0)"=u16 54321, "name"="CMD", "data"=T2 {"EXECUTE_SP"=FALSE, "ALARM_PRESS_DOWN_DUT"=FALSE, "ALARM_PRESS_DOWN_CHAMBER"=FALSE, "ALARM_PRESS_DOWN_DUT_CHAMBER"=TRUE, "FILING_DUT"=FALSE, "FILING_CHAMBER"=FALSE, "BLOCK"=FALSE, "PUMP_STATION_OFF"=FALSE, "Leak start"=FALSE, "Leak stop"=FALSE, "Drain"=FALSE} ("CMD REG"), "timeout (25000 ms)"=1000, "error in (no error)"=w98) -> ("error out"=w97:errorcluster)  [unwired: 5 in, 2 out]
          }
          event "AO 0", "AO 1": Value Change {
            n43 = event-data() -> ()  [unwired: 1 in, 6 out]
            n44 = Unbundle By Name(w114) -> ("amc"=w123:refnum<class "MessageAMC.lvclass">)
            n45 = call "Read SVW.vi"("GUI in"=w113) -> ("SharedVariableWrapper.lvclass"=w122:refnum<class "SharedVariableWrapper.lvclass">)  [unwired: 10 in]
            n46 = Build Array("AO 0", "AO 1") -> (w115:dbl[])
            n47 = call "ReadConfig.vi"("SharedVariableWrapper in"=w122) -> ("config"=w121:T5)  [unwired: 12 in, 2 out]
            n48 = Unbundle By Name(w121) -> ("ip"=w120:string)
            n49 = call "SendNetworkVariant.vi"("reference in"=w123, "receiver process"="STAND", "receiver host"=w120, "receiver port (0)"=u16 54321, "name"="SET_AOS", "data"=w115, "timeout (25000 ms)"=1000, "error in (no error)"=w112) -> ("error out"=w111:errorcluster)  [unwired: 5 in, 2 out]
          }
          event "+0,1", "-0,1", "=0": Value Change {
            n50 = event-data() -> ()  [unwired: 1 in, 6 out]
            n51 = case shown="True" "=0" {
              frame False {
              }
              frame True {
                n52 = property on="AO 0" class="Slide (strict)"("Val(Sgnl)"=0.0 ("Value (Signaling)")) -> ()  [unwired: 2 in, 2 out]
              }
            }
            n53 = case shown="True" "-0,1" {
              frame False {
              }
              frame True {
                n54 = property on="AO 0" class="Slide (strict)"() -> ("Value"=w138:dbl)  [unwired: 2 in, 2 out]
                n55 = Subtract(x=w138, y=0.1) -> (x-y=w137:dbl)
                n56 = property on="AO 0" class="Slide (strict)"("Val(Sgnl)"=w137) -> ()  [unwired: 2 in, 2 out]
              }
            }
            n57 = case shown="True" "+0,1" {
              frame False {
              }
              frame True {
                n58 = property on="AO 0" class="Slide (strict)"() -> ("Value"=w135:dbl)  [unwired: 2 in, 2 out]
                n59 = Add(x=w135, y=0.1) -> (x+y=w134:dbl)
                n60 = property on="AO 0" class="Slide (strict)"("Val(Sgnl)"=w134) -> ()  [unwired: 2 in, 2 out]
              }
            }
          }
        }
      }
      frame "---------- Core ----------" {
        n61 = call <vilib>:"Add State(s) to Queue__JKI_lib_State_Machine.vi"("State(s) in (\"\")"=w144) -> ("States Out"=w143:string)  [unwired: 14 in]
      }
      frame Default {
        w155 = 42 items=["No error", "Argument error", "Memory is full", "Out of zone", "End of file", "File already open", "Generic file I/O error", "File not found", "File permission error", "Disk is full", "Duplicate path", "Too many files open", "System feature not enabled", "Resource file not found", "Cannot add resource", "Resource not found", "Image not found", "Image memory error", "Pen does not exist", "Config type invalid", "Config token not found", "Config parse error", "Config memory error", "Bad external code format", "Bad external code offset", "External code not present", "Null window", "Destroy window error", "Null menu", "Print aborted", "Bad print record", "Print driver error", "Windows error during printing", "Memory error during printing", "Print dialog error", "Generic print error", "Invalid device refnum", "Device not found", "Device parameter error", "Device unit error", "Cannot open device", "Device call aborted", "Generic error", "Cancelled by user", "Object ID too low", "Object ID too high", "Object not in heap", "Unknown heap", "Unknown object (invalid DefProc)", "Unknown object (DefProc not in table)", "Message out of range", "Invalid (null) method", "Unknown message", "Manager call not supported", "Bad address", "Network operation in progress", "Network operation timed out", "Connection is busy", "Network attribute not supported", "Network error", "Address in use", "System out of memory", "Connection aborted", "Connection refused", "Not connected", "Already connected", "Connection closed", "Initialization error (interapplication manager)", "Bad occurrence", "Wait on unbound occurrence handler", "Occurrence queue overflow", "Datalog type conflict", "Unused", "Unrecognized type (interapplication manager)", "Memory corrupt", "Failed to make temporary DLL", "Old CIN version", "Drag socket not found", "Failed to load drop-object", "Failed to register OLE object", "Failed to release OLE object", "Format specifier type mismatch", "Unknown format specifier", "Too few format specifiers", "Too many format specifiers", "Scan failed", "Newer CIN version", "Error converting to variant", "Runtime menu error", "Password tampered", "Variant attribute not found", "Incompatible variant data type", "Event data is not available", "Event Store is not present", "Occurrence is not found", "Event Queue is not created", "Event info is not available", "Refnum passed is NULL", "Error retrieving Class GUID", "Error retrieving CoClass GUID", "Error retrieving TypeLib GUID.", "Bad built application magic bytes.", "Specific driver is different from the specific driver associated with the Logical Name.", "There is no session opened to the class driver.", "Max Error", "MAX - Error with config objects", "MAX - Error loading configuration", "MAX - Group not supported"]
        # "Current State"
        # "Do not delete, rename, or modify this frame.\n(this is used to capture unhandled states and typos)"
        # "Handle mistyped state name (developer tool)"
        n62 = Format Into String(format string="Software Exception: Unhandled State \"%s\"." ("message"), error in=w151, w146) -> (resulting string=w154:string, error out=w153:errorcluster)  [unwired: 1 in]
        n63 = call <vilib>:"Error Cluster From Error Code.vi"("show call chain? (False)"=TRUE, "error in (no error)"=w153, "error message (\"\")"=w154, "error code (0)"=w155) -> ("error out"=w152:errorcluster)  [unwired: 5 in]
        n64 = call <vilib>:"Add State(s) to Queue__JKI_lib_State_Machine.vi"("State(s) in (\"\")"=w150) -> ("States Out"=w149:string)  [unwired: 14 in]
      }
      frame "Initialize Core Data" {
        # "originally closed?"
        # "exe?"
        # "If panel starts closed or is an EXE, then close it when we exit"
        n65 = property class="VI"() -> ("FP.State"=w160:T3)  [unwired: 2 in, 2 out]
        n66 = property class="App"() -> ("App.Kind"=w166:T4)  [unwired: 2 in, 2 out]
        n67 = control-ref of="Current VI Reference"() -> (w161:refnum<vi>)
        n68 = Equal?(x=w160, y=T3."Closed" ("Front Panel Window:State")) -> (x = y?=w158:bool)
        n69 = Equal?(x=w166, y=T4."Run Time System" ("Application:Kind")) -> (x = y?=w164:bool)
        n70 = Or(x=w158, y=w164) -> (x .or. y?=w162:bool)
        n71 = Bundle By Name(cluster=w163, "Core.Current VI Reference"=w161, "Core.Close Panel on Exit?"=w162) -> (w168:T6)
        n72 = call <vilib>:"Add State(s) to Queue__JKI_lib_State_Machine.vi"("State(s) in (\"\")"=w170) -> ("States Out"=w169:string)  [unwired: 14 in]
      }
      frame "Error Handler" {
        # "Unhandled Error -- Display it"
        # "Handle any errors here.\nYou can also output any states to clean-up after errors occur"
        # "Clear error"
        n73 = call <vilib>:"General Error Handler.vi"("error in (no error)"=w173) -> ()  [unwired: 10 in, 5 out]
        n74 = call <vilib>:"Add State(s) to Queue__JKI_lib_State_Machine.vi"("State(s) in Front (\"\")"="/* Post Error States", "State(s) in (\"\")"=w177) -> ("States Out"=w176:string)  [unwired: 13 in]
      }
      frame "Exit" {
        n75 = Unbundle By Name(w180) -> ("amc"=w179:refnum<class "MessageAMC.lvclass">)
        n76 = call-dynamic "Destroy.vi"("reference in"=w179) -> ("error out"=w178:errorcluster)  [unwired: 17 in, 1 out]
        n77 = call <vilib>:"Clear Errors.vi"("error in (no error)"=w178) -> ()  [unwired: 5 in, 2 out]
        n78 = call <vilib>:"Add State(s) to Queue__JKI_lib_State_Machine.vi"("State(s) in (\"\")"=w185) -> ("States Out"=w184:string)  [unwired: 14 in]
      }
      frame "---------- Data ----------" {
        # "Do not put any code in this frame.\n(It is a separator no-op. You can make a copy of this frame to create a new Data frame)"
        n79 = call <vilib>:"Add State(s) to Queue__JKI_lib_State_Machine.vi"("State(s) in (\"\")"=w190) -> ("States Out"=w189:string)  [unwired: 14 in]
      }
      frame "Data: Initialize" {
        w197 = T7 {"Current VI Reference"=refnum, "Close Panel on Exit?"=FALSE}  # Core
        n80 = call "MessageAMC_Create.vi"("reference in"=refnum<class "MessageAMC.lvclass"> refnum, "error in (no error)"=w193, "message queue name"="GUI_TEST_CHNLS") -> ("amc"=w194:refnum<class "MessageAMC.lvclass">, "error out"=w192:errorcluster)  [unwired: 15 in]
        n81 = Bundle("Core"=w197, "amc"=w194) -> (w198:T6)  [unwired: 1 in]
      }
      frame "Data: Cleanup" {
        # "Cleanup any data and references, here.\n(this is called automatically, by the Macro: Exit)"
        n82 = Unbundle By Name(w201) -> ("Core.Current VI Reference"=w204:refnum<vi>)
        n83 = Close Reference(reference=w204, error in (no error)=w203) -> (error out=w202:errorcluster)
        n84 = call <vilib>:"Add State(s) to Queue__JKI_lib_State_Machine.vi"("State(s) in (\"\")"=w206) -> ("States Out"=w205:string)  [unwired: 14 in]
      }
      frame "---------- Events ----------" {
        # "Do not put any code in this frame.\n(It is a separator no-op. You can make a copy of this frame to create a new UI frame)"
        n85 = call <vilib>:"Add State(s) to Queue__JKI_lib_State_Machine.vi"("State(s) in (\"\")"=w211) -> ("States Out"=w210:string)  [unwired: 14 in]
      }
      frame "Events: Register" {
        n86 = call "Read stop event.vi"("GUI in"=w213) -> ("stop event"=w212:refnum<user-event>)  [unwired: 8 in, 2 out]
        n87 = register-events(error in=w214, w212) -> (reference out=w216:refnum<event-registration>, error out=w215:errorcluster)  [unwired: 1 in]
      }
      frame "Events: Unregister" {
        # "Do not put any code in this frame.\n(It is a separator no-op. You can make a copy of this frame to create a new UI frame)"
        n88 = Unregister For Events(event registration refnum=w221, error in=w220) -> (error out=w219:errorcluster)
        n89 = call <vilib>:"Add State(s) to Queue__JKI_lib_State_Machine.vi"("State(s) in (\"\")"=w224) -> ("States Out"=w223:string)  [unwired: 14 in]
      }
      frame "---------- UI ----------" {
        # "Do not put any code in this frame.\n(It is a separator no-op. You can make a copy of this frame to create a new UI frame)"
        n90 = call <vilib>:"Add State(s) to Queue__JKI_lib_State_Machine.vi"("State(s) in (\"\")"=w229) -> ("States Out"=w228:string)  [unwired: 14 in]
      }
      frame "UI: Initialize" {
      }
      frame "UI: Cursor Set" {
        # "Argument"
        # "Set and Unset Cursor Busy.\n(Usage: \"UI: Cursor Set >> Busy|Idle\")"
        n91 = case shown="\"Idle\", Default" w235 {
          tunnel: w237 -> [w242 w244]
          tunnel: [w241 w243] -> w236
          frame "Idle", Default {
            n92 = call <vilib>:"Unset Busy.vi"("error in (no error)"=w242) -> ("error out"=w241:errorcluster)  [unwired: 10 in]
          }
          frame "Busy" {
            n93 = call <vilib>:"Set Busy.vi"("error in (no error)"=w244) -> ("error out"=w243:errorcluster)  [unwired: 9 in, 1 out]
          }
        }
        n94 = call <vilib>:"Add State(s) to Queue__JKI_lib_State_Machine.vi"("State(s) in (\"\")"=w240) -> ("States Out"=w239:string)  [unwired: 14 in]
      }
      frame "UI: Front Panel State" {
        # "Argument"
        # "Set Front Panel Open or Closed\n(Usage: \"UI: Front Panel State >> Open|Close\")"
        n95 = Unbundle By Name(w248) -> ("Core.Current VI Reference"=w247:refnum<vi>)
        n96 = case shown="\"Minimize\", \"Minimized\"" w246 {
          tunnel: w250 -> [w258 w273 w284 w297 w310]
          tunnel: [w260 w274 w286 w299 w312] -> w249
          tunnel: w247 -> [w259 w271 w285 w298 w311]
          frame "Open", "Standard", Default {
            w253 = T3."Standard" ("State")
            n97 = property class="VI"(reference=w259, error in=w258) -> (reference out=w256:refnum<vi>, error out=w257:errorcluster, "FP.State"=w255:T3)
            n98 = Not Equal?(x=w255, y=w253) -> (x != y?=w254:bool)
            n99 = case shown="True" w254 {
              tunnel: [w264 w266] -> w260
              tunnel: w257 -> [w263 w266]
              tunnel: w256 -> [w262 _]
              tunnel: w253 -> [w261 _]
              frame True {
                n100 = invoke class="VI" method="FP.Open"(reference=w262, error in=w263, "Activate"=TRUE, "State"=w261) -> (error out=w264:errorcluster)  [unwired: 1 in, 4 out]
              }
              frame False {
              }
            }
          }
          frame "Close", "Closed" {
            n101 = property class="VI"(reference=w271, error in=w273) -> (reference out=w270:refnum<vi>, error out=w272:errorcluster, "FP.State"=w268:T3)
            n102 = Not Equal?(x=w268, y=T3."Closed" ("Front Panel Window:State")) -> (x != y?=w267:bool)
            n103 = case shown="True" w267 {
              tunnel: [w275 w278] -> w274
              tunnel: w272 -> [w275 w277]
              tunnel: w270 -> [_ w276]
              frame False {
              }
              frame True {
                n104 = invoke class="VI" method="FP.Close"(reference=w276, error in=w277) -> (error out=w278:errorcluster)  [unwired: 1 in, 2 out]
              }
            }
          }
          frame "Hidden", "Hide" {
            w279 = T3."Hidden" ("State")
            n105 = property class="VI"(reference=w285, error in=w284) -> (reference out=w282:refnum<vi>, error out=w283:errorcluster, "FP.State"=w281:T3)
            n106 = Not Equal?(x=w281, y=w279) -> (x != y?=w280:bool)
            n107 = case shown="True" w280 {
              tunnel: [w290 w291] -> w286
              tunnel: w283 -> [w289 w291]
              tunnel: w282 -> [w288 _]
              tunnel: w279 -> [w287 _]
              frame True {
                n108 = invoke class="VI" method="FP.Open"(reference=w288, error in=w289, "State"=w287) -> (error out=w290:errorcluster)  [unwired: 2 in, 4 out]
              }
              frame False {
              }
            }
          }
          frame "Minimize", "Minimized" {
            w292 = T3."Minimized" ("State")
            n109 = property class="VI"(reference=w298, error in=w297) -> (reference out=w295:refnum<vi>, error out=w296:errorcluster, "FP.State"=w294:T3)
            n110 = Not Equal?(x=w294, y=w292) -> (x != y?=w293:bool)
            n111 = case shown="True" w293 {
              tunnel: [w303 w304] -> w299
              tunnel: w296 -> [w302 w304]
              tunnel: w295 -> [w301 _]
              tunnel: w292 -> [w300 _]
              frame True {
                n112 = invoke class="VI" method="FP.Open"(reference=w301, error in=w302, "State"=w300) -> (error out=w303:errorcluster)  [unwired: 2 in, 4 out]
              }
              frame False {
              }
            }
          }
          frame "Maximize", "Maximized" {
            w305 = T3."Maximized" ("State")
            n113 = property class="VI"(reference=w311, error in=w310) -> (reference out=w308:refnum<vi>, error out=w309:errorcluster, "FP.State"=w307:T3)
            n114 = Not Equal?(x=w307, y=w305) -> (x != y?=w306:bool)
            n115 = case shown="True" w306 {
              tunnel: [w316 w317] -> w312
              tunnel: w309 -> [w315 w317]
              tunnel: w308 -> [w314 _]
              tunnel: w305 -> [w313 _]
              frame True {
                n116 = invoke class="VI" method="FP.Open"(reference=w314, error in=w315, "State"=w313) -> (error out=w316:errorcluster)  [unwired: 2 in, 4 out]
              }
              frame False {
              }
            }
          }
        }
        n117 = call <vilib>:"Add State(s) to Queue__JKI_lib_State_Machine.vi"("State(s) in (\"\")"=w252) -> ("States Out"=w251:string)  [unwired: 14 in]
      }
      frame "---------- Macro ----------" {
        # "Do not put any code in this frame.\n(It is a separator no-op. You can make a copy of this frame to create a new Macro frame)"
        n118 = call <vilib>:"Add State(s) to Queue__JKI_lib_State_Machine.vi"("State(s) in (\"\")"=w322) -> ("States Out"=w321:string)  [unwired: 14 in]
      }
      frame "Macro: Initialize" {
        n119 = call <vilib>:"Add State(s) to Queue__JKI_lib_State_Machine.vi"("State(s) in Front (\"\")"="Data: Initialize\nInitialize Core Data\nEvents: Register\nUI: Initialize\n// UI: Front Panel State >> Open\n\n\nAction: Read Config\nAction: Update Indicators\n", "State(s) in (\"\")"=w328) -> ("States Out"=w327:string)  [unwired: 13 in]
      }
      frame "Macro: Update" {
        n120 = call <vilib>:"Add State(s) to Queue__JKI_lib_State_Machine.vi"("State(s) in Front (\"\")"="Action: Update Indicators\nAction: Write Config", "State(s) in (\"\")"=w334) -> ("States Out"=w333:string)  [unwired: 13 in]
      }
      frame "Macro: Exit" {
        # "Exit Macro\n(This is called once, when the VI exits)"
        n121 = Unbundle By Name(w343) -> ("Core.Close Panel on Exit?"=w342:bool)
        n122 = Select(t="UI: Front Panel State >> Close", s=w342, f="") -> (s? t:f=w339:string)
        n123 = call <vilib>:"Add State(s) to Queue__JKI_lib_State_Machine.vi"("State(s) in Front (\"\")"="Action: Write Config", "State(s) in (\"\")"=w339, "State(s) at Back (\"\")"="Data: Cleanup\nEvents: Unregister\nExit") -> ("States Out"=w337:string)  [unwired: 12 in]
        n124 = call <vilib>:"Add State(s) to Queue__JKI_lib_State_Machine.vi"("State(s) in Front (\"\")"=w337, "State(s) in (\"\")"=w346) -> ("States Out"=w345:string)  [unwired: 13 in]
      }
      frame "---------- Action ----------" {
      }
      frame "Action: Read Config" {
        n125 = call <vilib>:"Add State(s) to Queue__JKI_lib_State_Machine.vi"("State(s) in (\"\")"=w351) -> ("States Out"=w352:string)  [unwired: 14 in]
      }
      frame "Action: Write Config" {
      }
      frame "Action: Update Indicators" {
      }
      frame "Action: Update Channels TBL" {
      }
    }
  }
  n126 = while {
    tunnel: w3 -> [w384]
    tunnel: w2 -> [w377]
    stop <- "stop" stop-if-true
    n127 = stacked-sequence {
      tunnel: w384 -> [w400 w470 w473 w487 w531 w541]
      tunnel: [w411 _ _ _ _ _] -> w380
      tunnel: [_ w439 _ _ _ _] -> w381
      tunnel: [_ _ _ _ w530 _] -> w382
      tunnel: [_ _ _ _ _ w540] -> w383
      tunnel: w377 -> [_ _ _ _ w528 w538]
      tunnel: [w401 _ _ _ _ _] -> w376
      tunnel: [_ _ w471 _ _ _] -> w375
      tunnel: [_ _ _ w484 _ _] -> w374
      tunnel: [_ _ _ w481 _ _] -> w373
      tunnel: [_ _ _ w480 _ _] -> w372
      tunnel: [w388 _ _ _ _ _] -> w371
      tunnel: [w387 _ _ _ _ _] -> w369
      frame #0 {
        w406 = "CALIBRATION_DATA"  # VAR
        n128 = control-ref of="AI 5"() -> (w417:refnum<vi>)
        n129 = control-ref of="AI 6"() -> (w416:refnum<vi>)
        n130 = control-ref of="AI 7"() -> (w415:refnum<vi>)
        n131 = control-ref of="AI 8"() -> (w414:refnum<vi>)
        n132 = control-ref of="AI 9"() -> (w413:refnum<vi>)
        n133 = control-ref of="AI 10"() -> (w412:refnum<vi>)
        n134 = control-ref of="AI_0"() -> (w399:refnum<vi>)
        n135 = control-ref of="AI1"() -> (w398:refnum<vi>)
        n136 = control-ref of="AI_2"() -> (w397:refnum<vi>)
        n137 = control-ref of="AI3"() -> (w396:refnum<vi>)
        n138 = control-ref of="AI4"() -> (w395:refnum<vi>)
        n139 = Build Array(w399, w398, w397, w396, w395) -> (w391:refnum<vi>[])
        n140 = call "Read.vim"("SharedVariableWrapper in"=w400, "name"=w406, "DataType"=T8 {"Channels"=[], "Scales"=[]} ("CalibrationData")) -> ("data out"=w404:T8, "error out"=w402:errorcluster)  [unwired: 6 in, 5 out]
        n141 = call "Read.vim"("SharedVariableWrapper in"=w400, "name"="AI_ARRAY", "DataType"=T12 [] ("AI_Data_Array")) -> ("connected"=w420:bool, "data out"=w410:T12, "error out"=w419:errorcluster)  [unwired: 6 in, 4 out]
        n142 = Build Array(w417, w416, w415, w414, w413, w412) -> (w407:refnum<vi>[])
        n143 = Unbundle By Name(w404) -> ("Channels"=w403:T9[])
        n144 = Build Array (concatenate)(w391, w407) -> (w392:refnum<vi>[])
        n145 = call <vilib>:"Clear Errors.vi"("error in (no error)"=w419) -> ("error out"=w418:errorcluster)  [unwired: 5 in, 1 out]
        n146 = Array Subset(array=w403, index=5) -> (w394:T9[])  [unwired: 1 in]
        n147 = Index Array(array=w410, index #1=5 ("index")) -> (element #1=w389:T13, element #2=w409:T13, element #3=w390:T13)  [unwired: 2 in]
        n148 = for {
          tunnel: w420 -> [w431]
          tunnel: w410 -> [w432]
          shift-right: [w433] -> w411
          shift-left: w418 -> [w434]
          tunnel: w392 -> [w428] mode=indexing
          i -> [w429]
          n149 = Index Array(array=w432, index=w429) -> (element=w430:T13)
          n150 = call "UpdateNumericWithScale.vi"("NumericWithScale in"=w428, "connect"=w431, "AI_Data"=w430, "error in (no error)"=w434) -> ("error out"=w433:errorcluster)  [unwired: 11 in]
        }
        n151 = for {
          tunnel: w407 -> [w427] mode=indexing
          tunnel: w394 -> [w426] mode=indexing
          shift-right: [w424] -> w401
          shift-left: w402 -> [w423]
          n152 = Unbundle By Name(w426) -> ("AI Ranges"=w425:T10)
          n153 = call "Set Color Zones.vim"("reference"=w427, "AI Ranges"=w425, "error in (no error)"=w423) -> ("error out"=w424:errorcluster)  [unwired: 12 in]
        }
        n154 = Unbundle By Name(w409) -> ("Stat Data.scl mean 1Hz"=w388:dbl)
        n155 = Unbundle By Name(w390) -> ("Stat Data.scl mean 1Hz"=w387:dbl)
        n156 = Unbundle By Name(w389) -> ()  [unwired: 1 out]
      }
      frame #1 {
        n157 = call "Read.vim"("SharedVariableWrapper in"=w470, "name"="DI_ARRAY", "DataType"=bool[] []) -> ("data out"=w440:bool[], "error out"=w439:errorcluster)  [unwired: 6 in, 5 out]
        n158 = Index Array(array=w440) -> (element #1=→"DI 0":bool, element #2=→"DI 1":bool, element #3=→"DI 2":bool, element #4=→"DI 3":bool, element #5=→"DI 4":bool, element #6=→"DI 5":bool, element #7=→"DI 6":bool, element #8=→"DI 7":bool, element #9=→"DI 8":bool, element #10=→"DI 9":bool, element #11=→"DI 10":bool, element #12=→"DI 11":bool, element #13=→"DI 12":bool, element #14=→"DI 13":bool, element #15=→"DI 14":bool, element #16=→"DI 15":bool, element #17=→"DI 16":bool, element #18=→"DI 17":bool, element #19=→"DI 18":bool, element #20=→"DI 19":bool, element #21=→"DI 20":bool, element #22=→"DI 21":bool, element #23=→"DI 22":bool, element #24=→"DI 23":bool, element #25=→"DI 24":bool, element #26=→"DI 25":bool, element #27=→"DI 26":bool, element #28=→"DI 27":bool, element #29=→"DI 28":bool, element #30=→"DI 29":bool, element #31=→"DI 30":bool)  [unwired: 31 in]
      }
      frame #2 {
        n159 = call "Read.vim"("SharedVariableWrapper in"=w473, "name"="VLV_44_1_STATE", "DataType"=valveState."Unknown" ("valveState")) -> ("data out"=→"data out":T1, "error out"=w472:errorcluster)  [unwired: 6 in, 5 out]
        n160 = call "Read.vim"("SharedVariableWrapper in"=w473, "name"="VLV_44_2_STATE", "DataType"=valveState."Unknown" ("valveState"), "error in (no error)"=w472) -> ("data out"=→"data out 2":T1, "error out"=w471:errorcluster)  [unwired: 5 in, 5 out]
      }
      frame #3 {
        w485 = T13 {"Stat Data"={"raw mean"=0.0, "scl mean"=0.0, "raw mean 1Hz"=0.0, "scl mean 1Hz"=0.0}, "OutOfRangeMax"=FALSE, "OutOfRangeMin"=FALSE, "HIHI"=FALSE, "HI"=FALSE, "LO"=FALSE, "LOLO"=FALSE} ("AI_Data")
        n161 = call "Read.vim"("SharedVariableWrapper in"=w487, "name"="P_CHMBR_MB", "DataType"=w485) -> ("data out"=w482:T13, "error out"=w486:errorcluster)  [unwired: 6 in, 5 out]
        n162 = call "Read.vim"("SharedVariableWrapper in"=w487, "name"="P_DUT_MB", "DataType"=w485, "error in (no error)"=w486) -> ("data out"=w483:T13, "error out"=w484:errorcluster)  [unwired: 5 in, 5 out]
        n163 = Unbundle By Name(w482) -> ("Stat Data.scl mean 1Hz"=w480:dbl)
        "P_CHMBR_MB" <- w480
        n164 = Unbundle By Name(w483) -> ("Stat Data.scl mean 1Hz"=w481:dbl)
        "P_DUT_MB" <- w481
      }
      frame #4 {
        n165 = call "GetSheredData.vi"("reference in"=w528) -> ("data"=w529:T16)  [unwired: 12 in, 2 out]
        n166 = Unbundle By Name(w529) -> ("WindowsState"=w493:T15)
        n167 = Not Equal?(x=w493, y=WindowsState."Opened") -> (x != y?=w490:bool)
        n168 = control-ref of="DO 24"() -> (w495:refnum<vi>)
        n169 = control-ref of="DO 25"() -> (w494:refnum<vi>)
        n170 = control-ref of="DO 0"() -> (w513:refnum<vi>)
        n171 = control-ref of="DO 1"() -> (w509:refnum<vi>)
        n172 = control-ref of="DO 2"() -> (w514:refnum<vi>)
        n173 = control-ref of="DO 3"() -> (w510:refnum<vi>)
        n174 = control-ref of="DO 4"() -> (w511:refnum<vi>)
        n175 = control-ref of="DO 5"() -> (w512:refnum<vi>)
        n176 = control-ref of="DO 6"() -> (w515:refnum<vi>)
        n177 = control-ref of="DO 7"() -> (w516:refnum<vi>)
        n178 = control-ref of="DO 8"() -> (w517:refnum<vi>)
        n179 = control-ref of="DO 9"() -> (w518:refnum<vi>)
        n180 = control-ref of="DO 10"() -> (w519:refnum<vi>)
        n181 = control-ref of="DO 11"() -> (w520:refnum<vi>)
        n182 = control-ref of="DO 12"() -> (w521:refnum<vi>)
        n183 = control-ref of="DO 13"() -> (w522:refnum<vi>)
        n184 = control-ref of="DO 14"() -> (w523:refnum<vi>)
        n185 = control-ref of="DO 15"() -> (w524:refnum<vi>)
        n186 = control-ref of="DO 16"() -> (w525:refnum<vi>)
        n187 = control-ref of="DO 17"() -> (w502:refnum<vi>)
        n188 = control-ref of="DO 18"() -> (w501:refnum<vi>)
        n189 = control-ref of="DO 19"() -> (w500:refnum<vi>)
        n190 = control-ref of="DO 20"() -> (w499:refnum<vi>)
        n191 = control-ref of="DO 21"() -> (w498:refnum<vi>)
        n192 = control-ref of="DO 22"() -> (w497:refnum<vi>)
        n193 = control-ref of="DO 23"() -> (w496:refnum<vi>)
        n194 = call "Read.vim"("SharedVariableWrapper in"=w531, "name"="DO_ARRAY", "DataType"=bool[] [] ("appended array")) -> ("connected"=w503:bool, "data out"=w507:bool[], "error out"=w506:errorcluster)  [unwired: 6 in, 4 out]
        n195 = Build Array(w513, w509, w514, w510, w511, w512, w515, w516, w517, w518, w519, w520, w521, w522, w523, w524, w525, w502, w501, w500, w499, w498, w497, w496, w495, w494) -> (w504:refnum<vi>[])
        n196 = call "Is Value Changed.vim"("value"=w507) -> ("changed or first call?"=w508:bool)
        n197 = Or(x=w508, y=w490) -> (x .or. y?=w491:bool)
        n198 = case shown="True" w491 {
          tunnel: w504 -> [_ w536]
          tunnel: w507 -> [_ w535]
          tunnel: w506 -> [w532 w534]
          tunnel: [w532 w533] -> w505
          frame False {
          }
          frame True {
            n199 = call "SetValueWithDisable.vim"("error in (no error)"=w534, "value"=w535, "Ctl Refnum"=w536) -> ("error out"=w533:errorcluster)  [unwired: 8 in]
          }
        }
        n200 = call "DisableControls.vim"("error in (no error)"=w505, "enable"=w503, "Array"=w504) -> ("error out"=w530:errorcluster)  [unwired: 8 in]
      }
      frame #5 {
        n201 = call "GetSheredData.vi"("reference in"=w538) -> ("data"=w539:T16)  [unwired: 12 in, 2 out]
        n202 = Unbundle By Name(w539) -> ("WindowsState"=w537:T15)
        n203 = case shown="Default" w537 {
          tunnel: w541 -> [_ w554]
          tunnel: [_ w553] -> w540
          frame "Opened" {
          }
          frame Default {
            n204 = call "Read.vim"("SharedVariableWrapper in"=w554, "name"="AO_ARRAY", "DataType"=dbl[] [] ("appended array")) -> ("connected"=w542:bool, "data out"=w548:dbl[], "error out"=w547:errorcluster)  [unwired: 6 in, 4 out]
            n205 = control-ref of="AO 1"() -> (w546:refnum<vi>)
            n206 = control-ref of="AO 0"() -> (w545:refnum<vi>)
            n207 = call "Is Value Changed.vim"("value"=w548) -> ("changed or first call?"=w549:bool)
            n208 = Build Array(w545, w546) -> (w550:refnum<vi>[])
            n209 = case shown="True" w549 {
              tunnel: w550 -> [w555 w557]
              tunnel: w548 -> [_ w560]
              tunnel: w547 -> [w556 w559]
              tunnel: [w556 w558] -> w544
              tunnel: [w555 w557] -> w543
              frame False {
              }
              frame True {
                n210 = call "SetValueWithDisable.vim"("error in (no error)"=w559, "value"=w560, "Ctl Refnum"=w557) -> ("error out"=w558:errorcluster)  [unwired: 8 in]
              }
            }
            n211 = call "DisableControls.vim"("error in (no error)"=w544, "enable"=w542, "Array"=w543) -> ("error out"=w553:errorcluster)  [unwired: 8 in]
          }
        }
      }
    }
    n212 = Bundle("scl mean 1Hz"=w373, "scl mean 1Hz"=w371) -> (→"DUT":cluster{"scl mean 1Hz":dbl, "scl mean 1Hz":dbl})  [unwired: 1 in]
    n213 = Bundle("scl mean 1Hz"=w372, "scl mean 1Hz"=w369) -> (→"CHMBR":cluster{"scl mean 1Hz":dbl, "scl mean 1Hz":dbl})  [unwired: 1 in]
    n214 = Merge Errors(w374, w376, w383, w382, w381, w380, w375) -> (w379:errorcluster)
    n215 = Wait Until Next ms Multiple(millisecond multiple=u32 100) -> ()  [unwired: 1 out]
    n216 = Unbundle By Name(w379) -> ("status"=→"Connect":bool)
  }
  n217 = flat-sequence {
    tunnel: w1 -> [w562]
    frame #0 {
      n218 = local write "stop"(TRUE ("stop")) -> ()
      "error out" <- w562
    }
  }
  n219 = flat-sequence {
    tunnel: w1 -> [_]
    frame #0 {
    }
  }
